vi "Demo Main_before_improvements.vi"() -> ()   [LabVIEW 2022 SP3]
uses:
  C:/Users/Public/OneDrive/Desktop/PMT program/SampleCodeLabView/Kinesis_with_LabVIEW_Examples_LV12 - v3/Thorlabs.MotionControl.Controls.dll
  Kinesis_with_LabVIEW_Examples_LV12 - v3/Thorlabs.MotionControl.Controls.dll
  C:/Users/Public/OneDrive/Desktop/PMT program/SampleCodeLabView/Kinesis_with_LabVIEW_Examples_LV12 - v3/ThorLabs.MotionControl.KCube.DCServoCLI.dll
  Kinesis_with_LabVIEW_Examples_LV12 - v3/ThorLabs.MotionControl.KCube.DCServoCLI.dll
  <vilib>/Utility/file.llb/Write Delimited Spreadsheet (I64).vi
  <vilib>/Utility/file.llb/Write Delimited Spreadsheet (string).vi
  <vilib>/Analysis/NI_AALBase.lvlib
  <vilib>/Utility/file.llb/Write Delimited Spreadsheet (DBL).vi
  Logo.ctl
panel:
  out "ESD":i32=10000 caption="Steps\nAdded/Removed"
  in  "ES":i32 caption="Add /Remove \nSteps"
  out "Sweep Graph":u32[](graph)
  out "SM":i32 caption="Sweep\nMean"
  out "SN":i32 caption="Current Sweep Iteration"
  out "SND":i32 caption="Total No. of Sweeps"
  in  "Auto-Sweep":bool
  in  "P8":bool
  out "PC":i32 caption="Current \nPosition"
  out "WTD":i32=10000 caption="Wait Time (ms)\nRead Data"
  out "EPD":i32 caption="End Position\nRead Data"
  out "SPD":i32 caption="Start Position\nRead Data"
  out "SSD":i32 caption="Step Size\nRead Data"
  in  "SP":i32 caption="Start Position (degrees)\n Set Data"
  in  "WT":i32=10000 caption="Wait Time (ms)\n Set Data"
  in  "EP":i32 caption="End Position (degrees)\n Set Data"
  in  "P7":bool
  in  "SS":i32 caption="Step Size (degrees)\nSet Data"
  in  "Motor Controller\nSerialNumber":string="27261255"
  in  "KCubeDCServoControl":refnum<k24>(container)
  in  "Export":bool
  out "DB":u32[](array[numeric])
  out "OVL":bool caption="LED ON : Over Rang Data"
  out "OLD":i32
  out "GN":i32 caption="Gate Number"
  in  "Correction":bool
  in  "Logo":T1
  out "Graph":u32[](graph)
  in  "Stop":bool
  in  "Start":bool
  in  "P6":bool
  out "RND":i32 caption="Read Number\nRead Data"
  in  "P5":bool
  in  "RN":i32=100 caption="Read Number\nSet Data"
  out "PowerD":i32 caption="Power\nRead Data"
  out "ITD":i32 caption="Internal Time\nRead Data"
  in  "P4":bool
  in  "P3":bool
  in  "IT":i32=100 caption="Internal Time\nSet Data"
  in  "P2":bool
  out "Handle Number":i32
  in  "P1":bool caption="Switch\nPower OFF/Power ON"
  in  "EXIT":bool
  # "pmt serial: 30430219"
  # "data array isn't being emptied after each sweep...?"
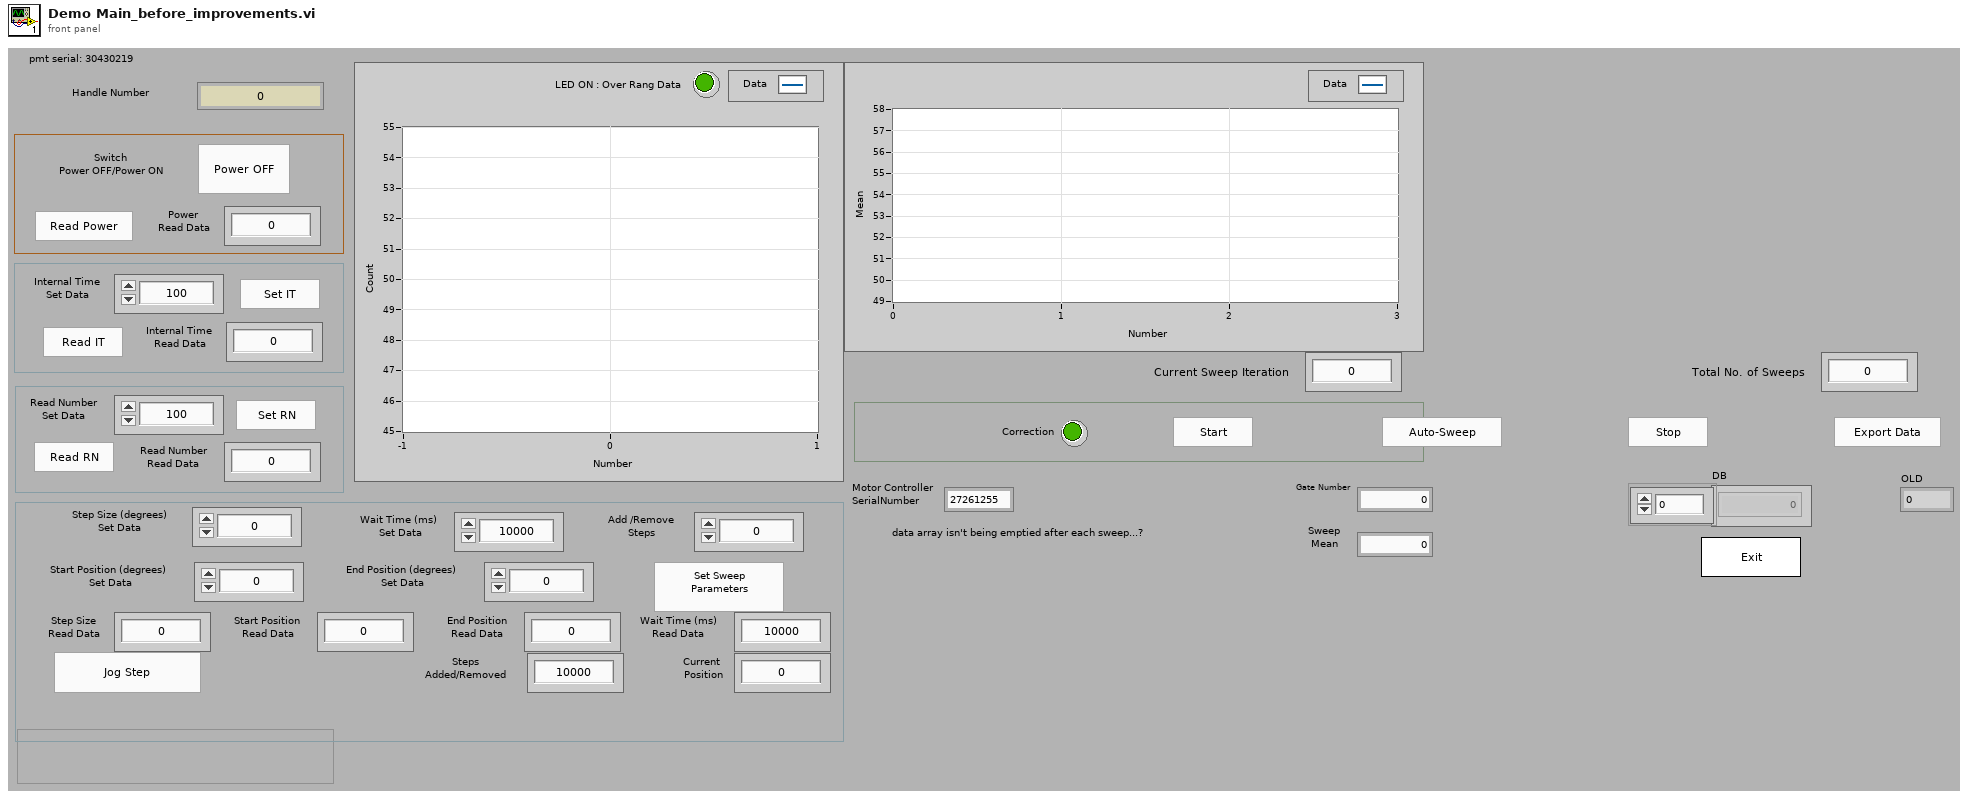
[diagram p1: front panel]
types:
  T1 = typedef "Logo.ctl" = bool
  T2 = enum8{"Enabled", "Disabled", "Disabled and Grayed Out"}
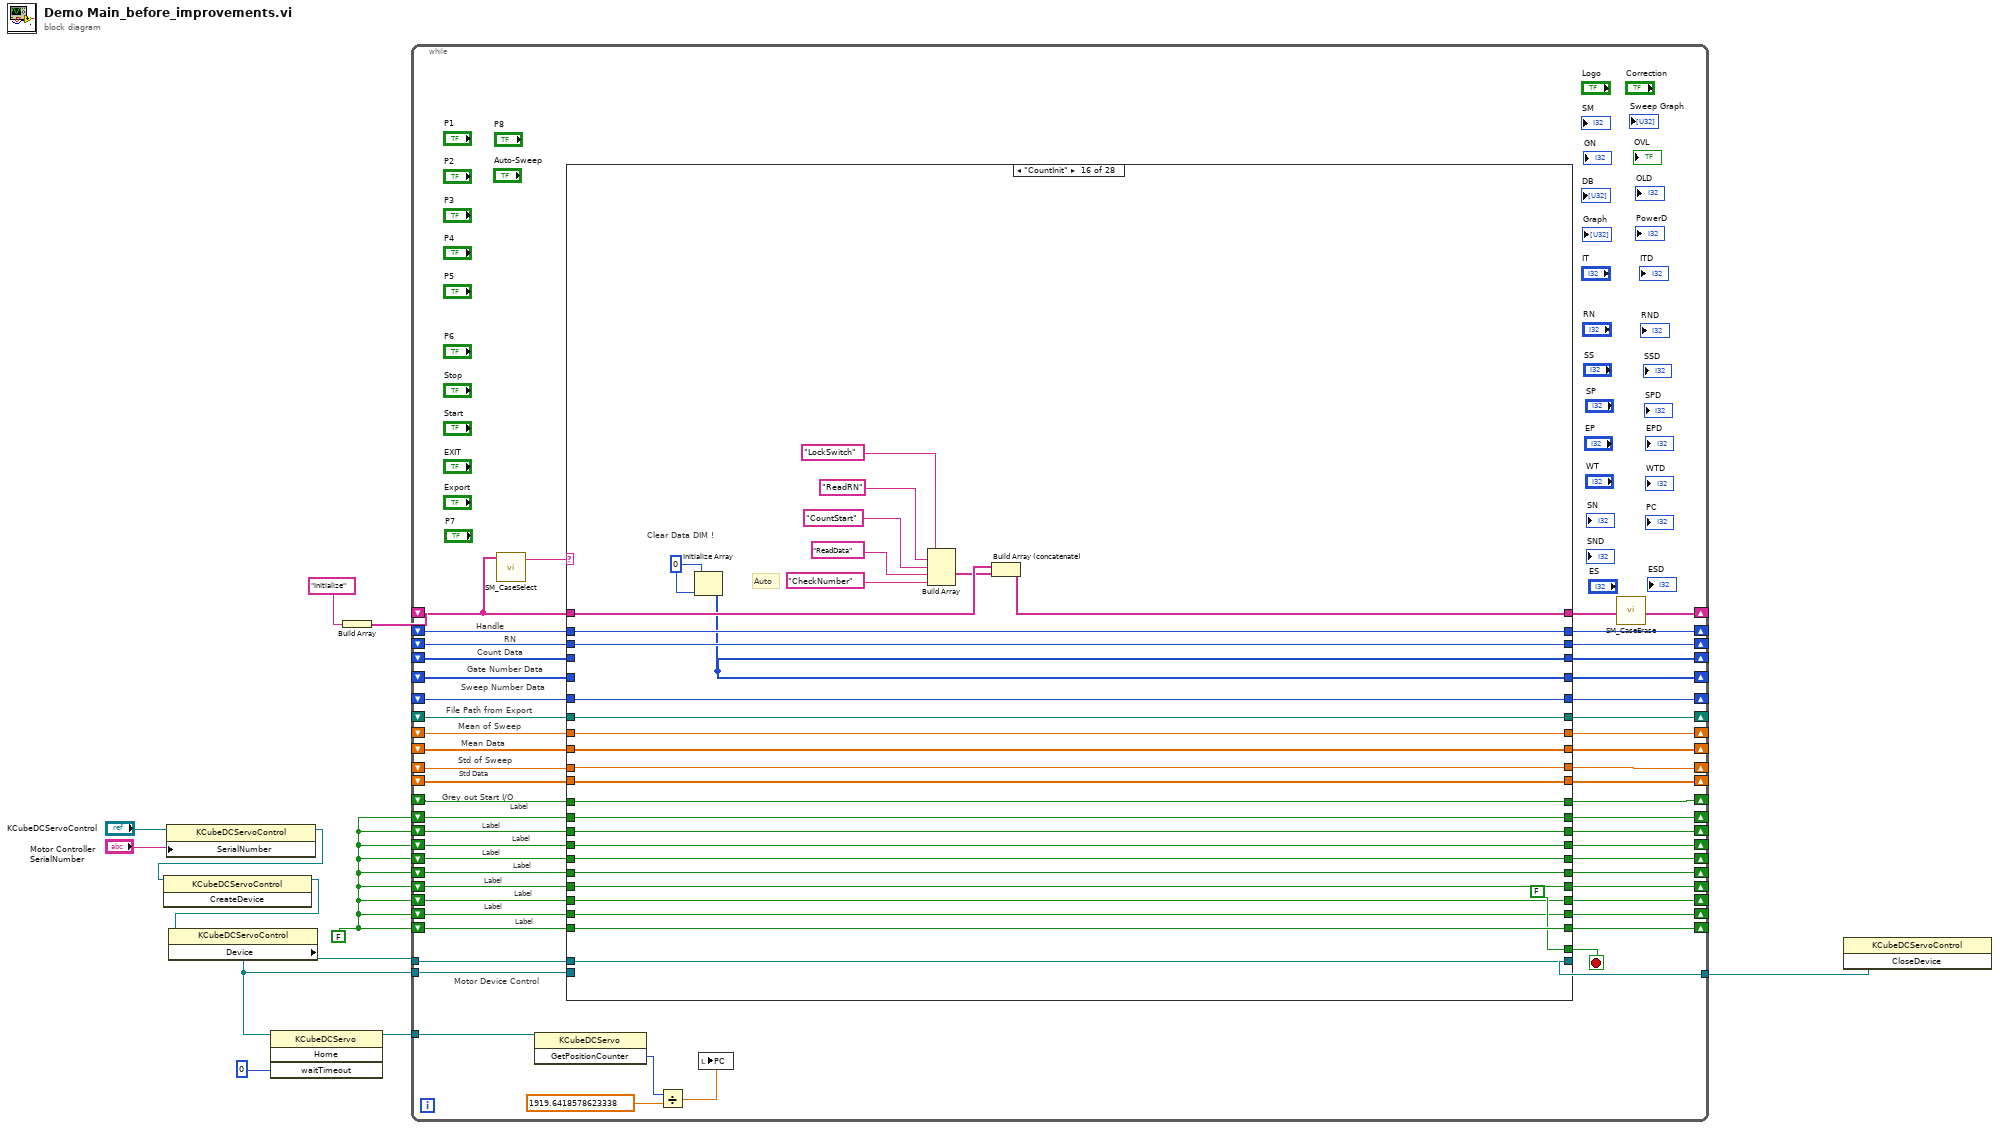
[diagram p0: block diagram]
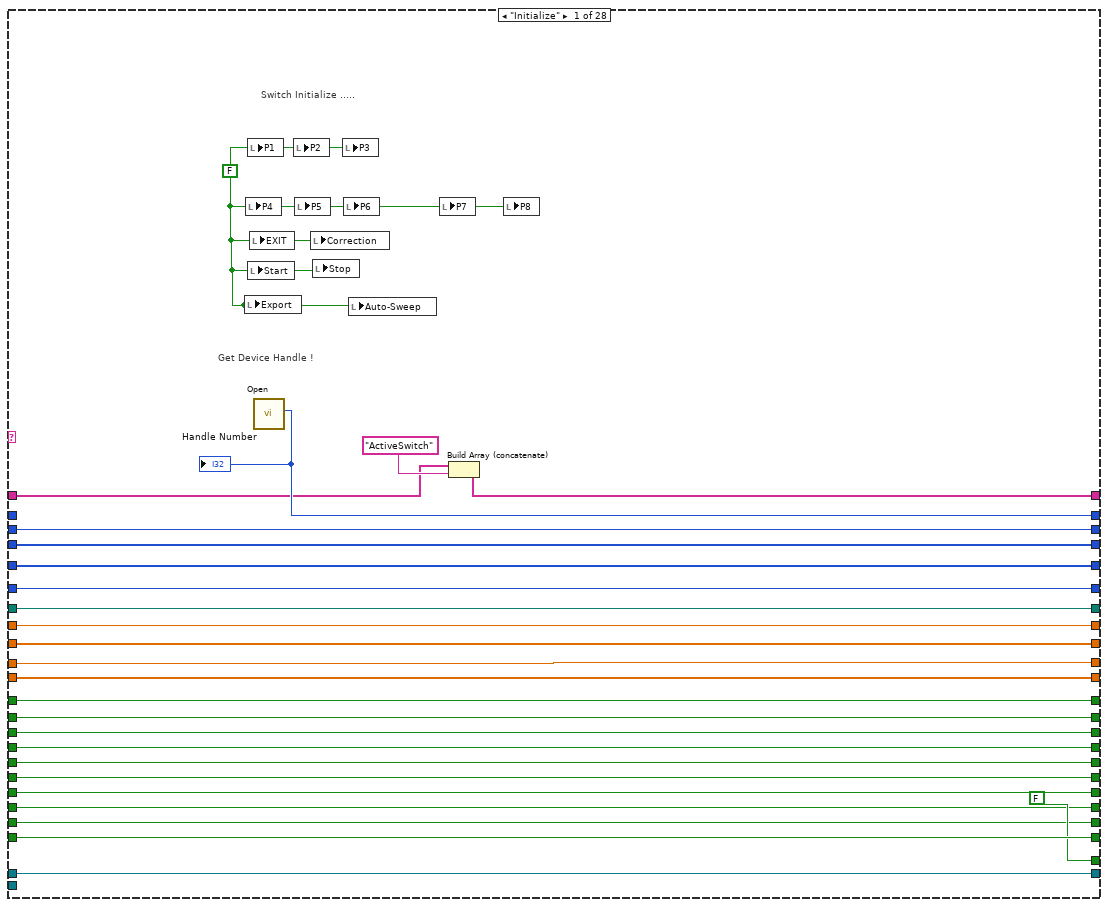
[diagram p2: hidden frame]
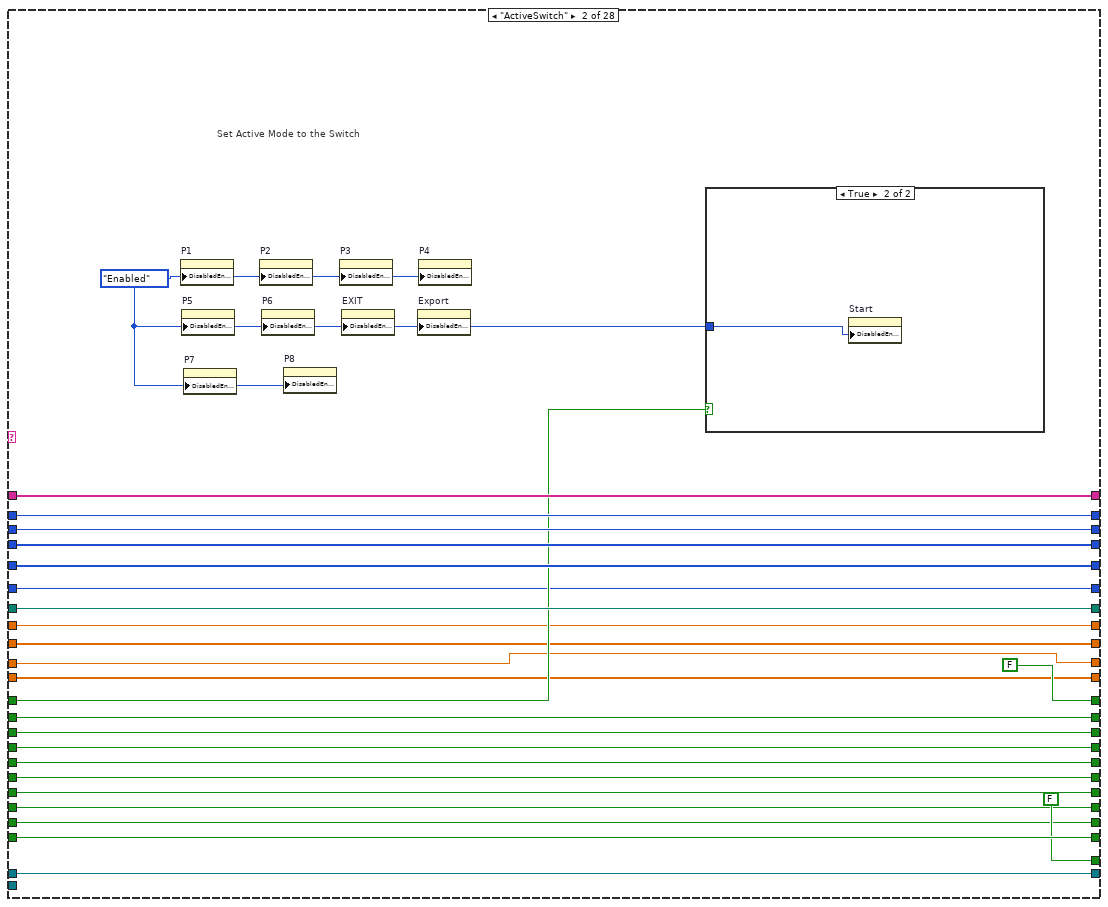
[diagram p3: hidden frame]
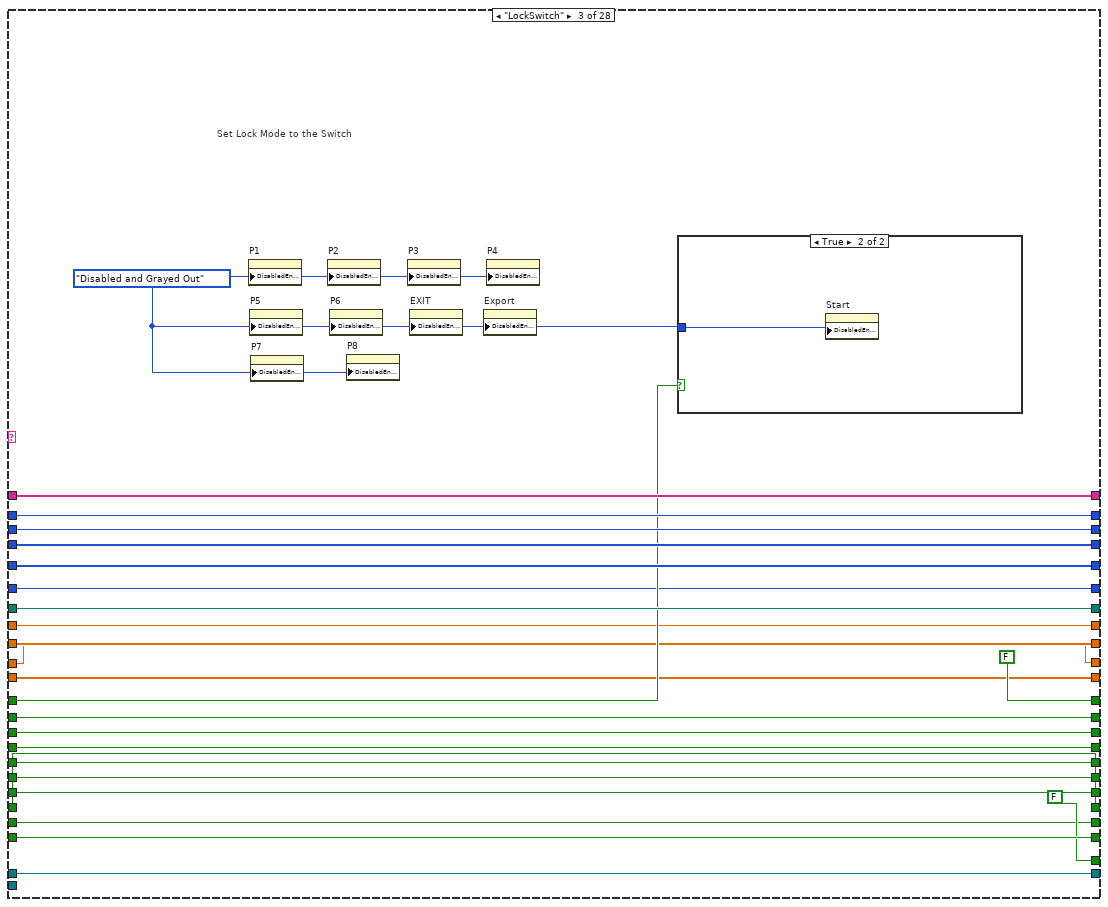
[diagram p5: hidden frame]
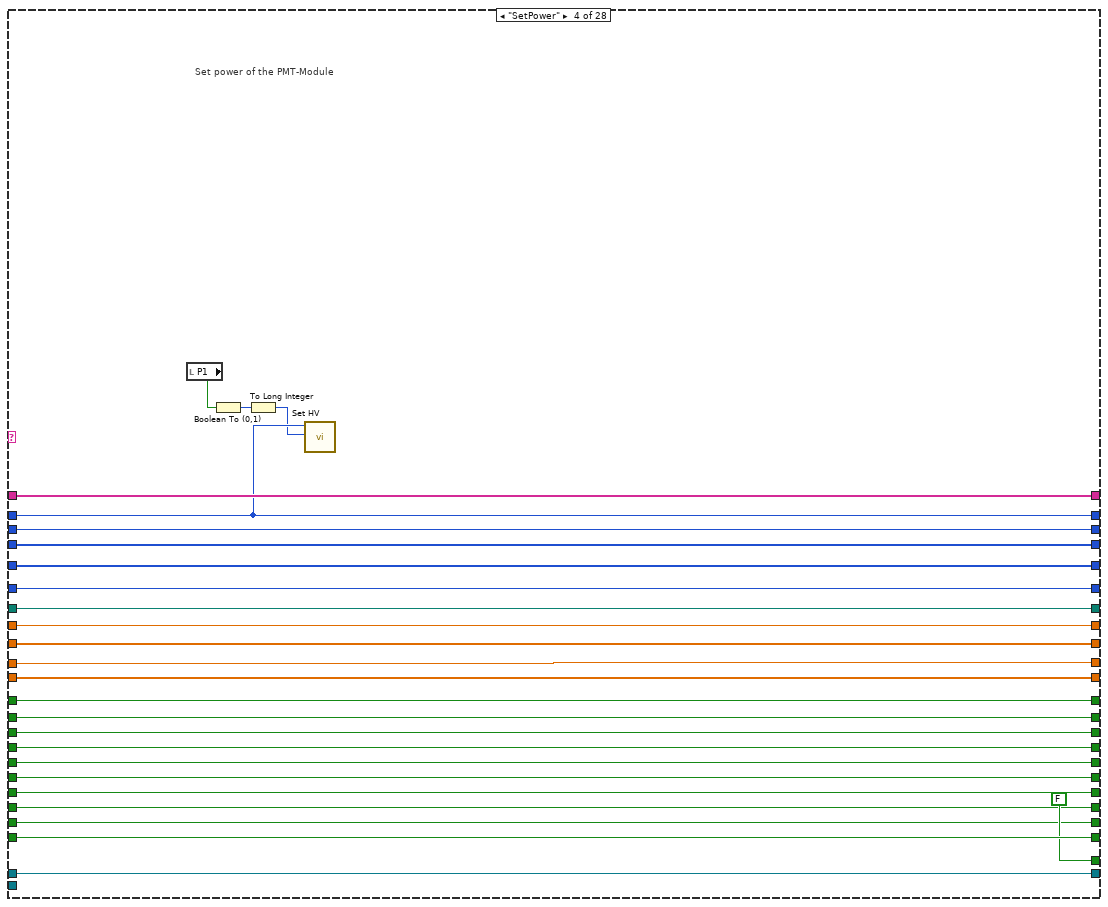
[diagram p7: hidden frame]
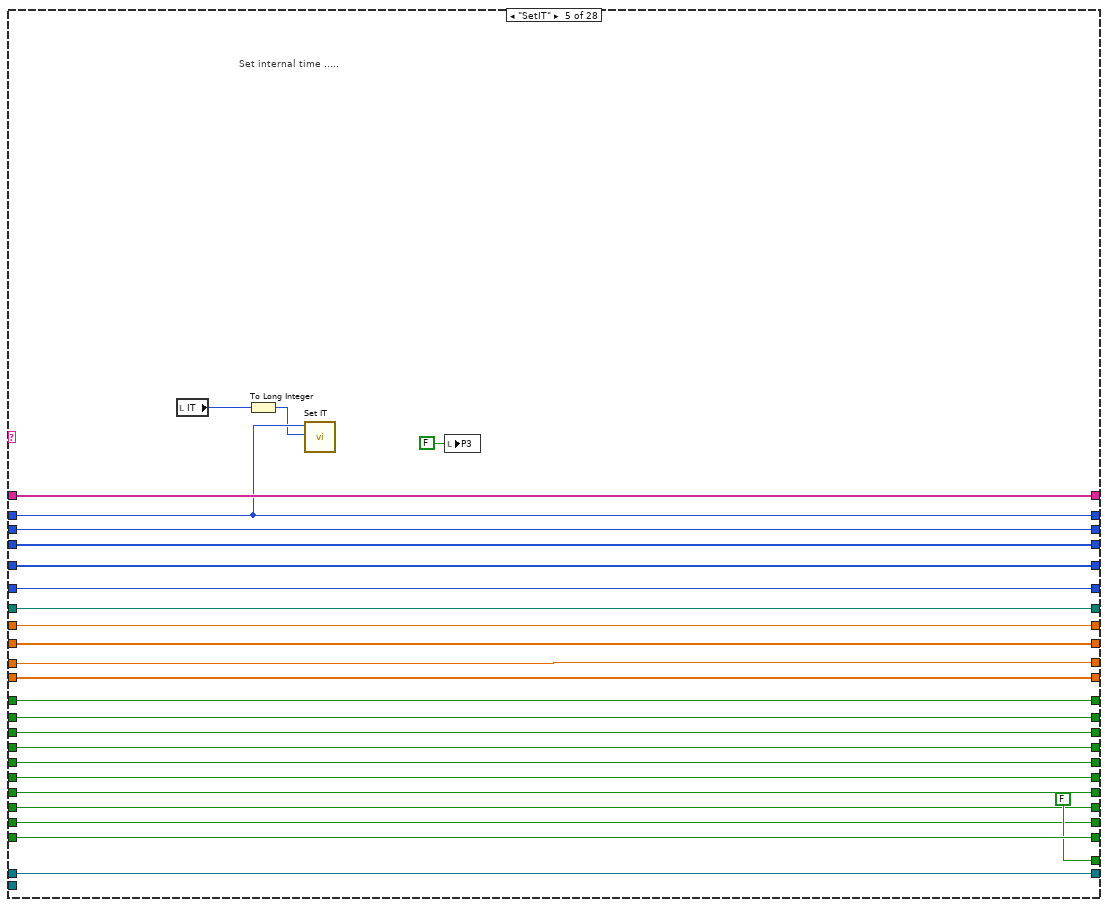
[diagram p8: hidden frame]
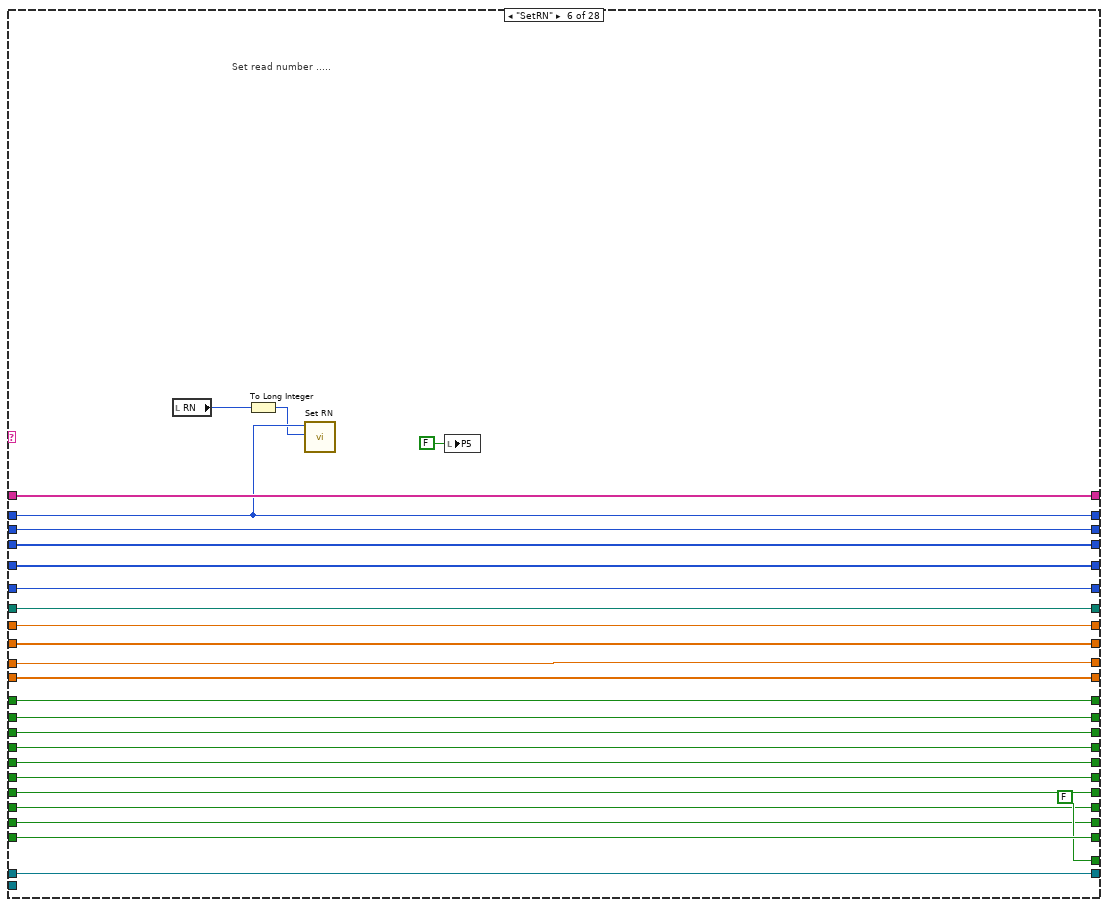
[diagram p9: hidden frame]
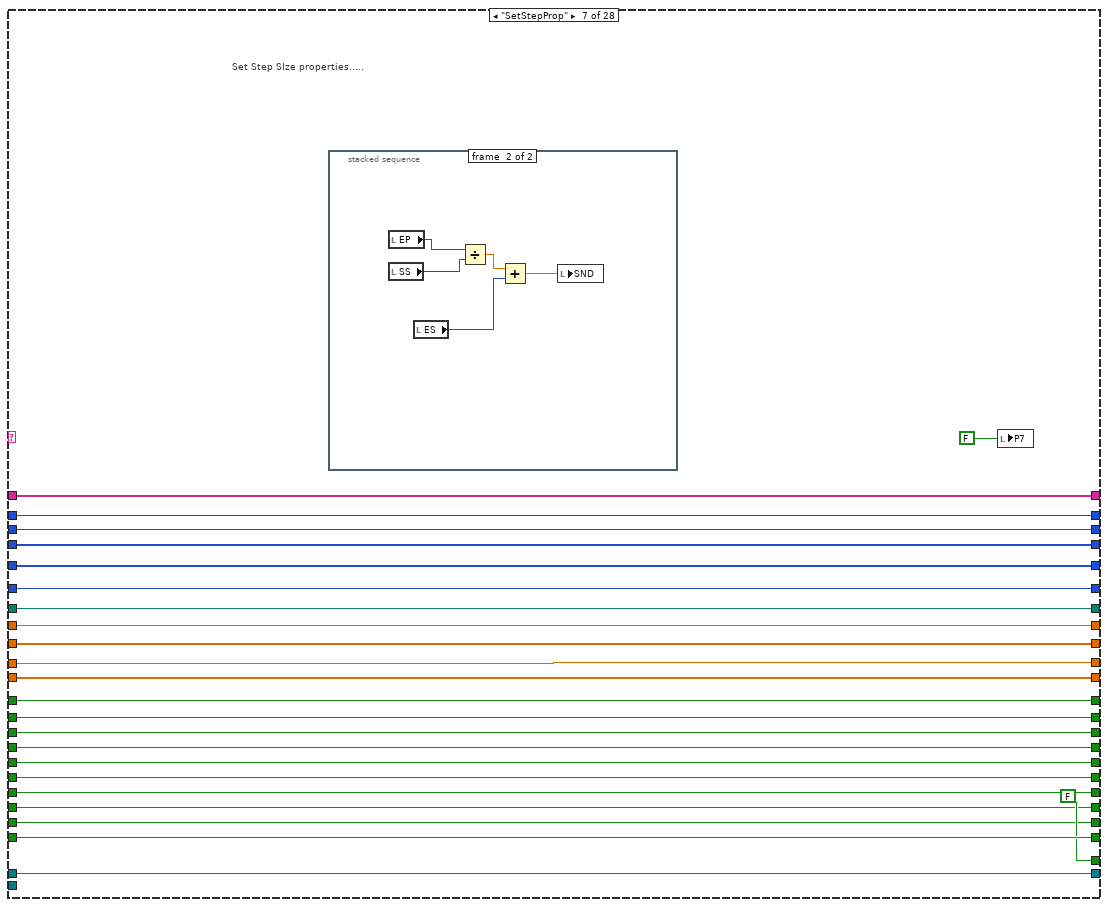
[diagram p10: hidden frame]
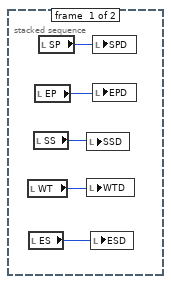
[diagram p11: hidden frame]
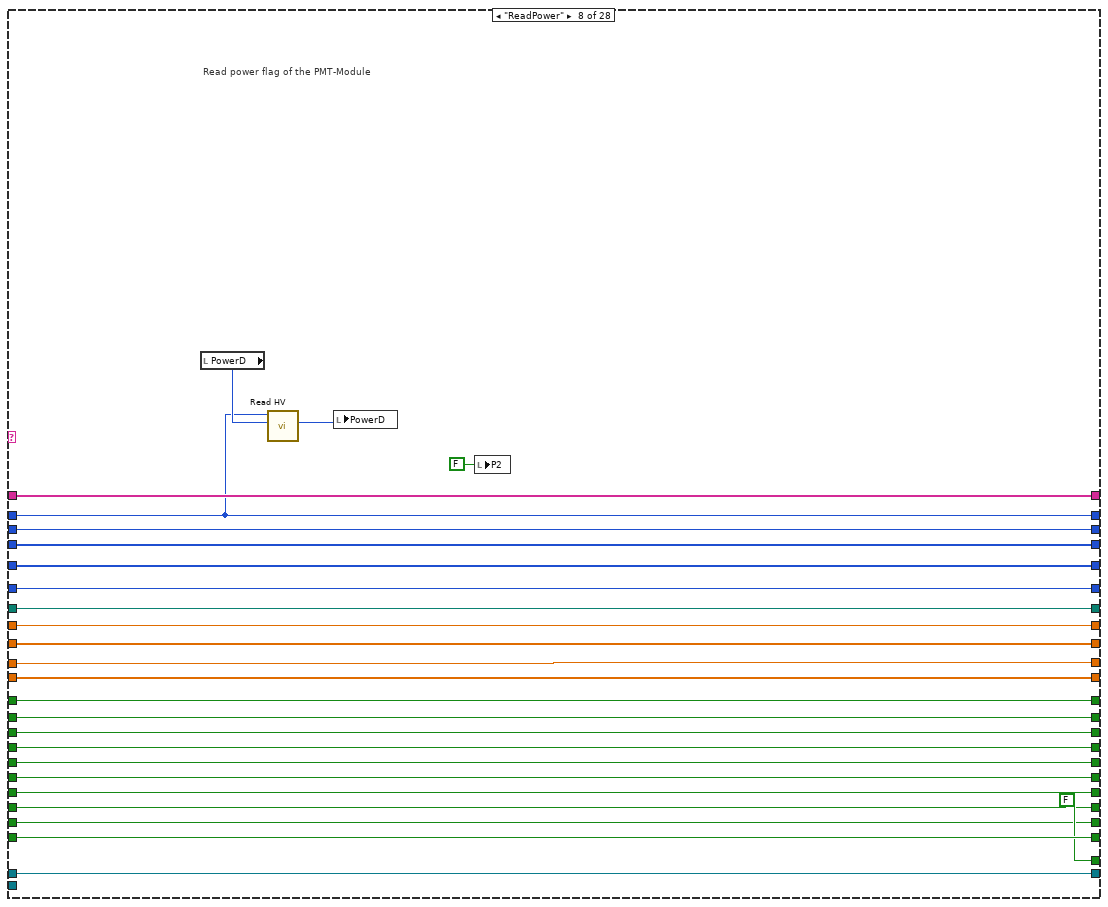
[diagram p12: hidden frame]
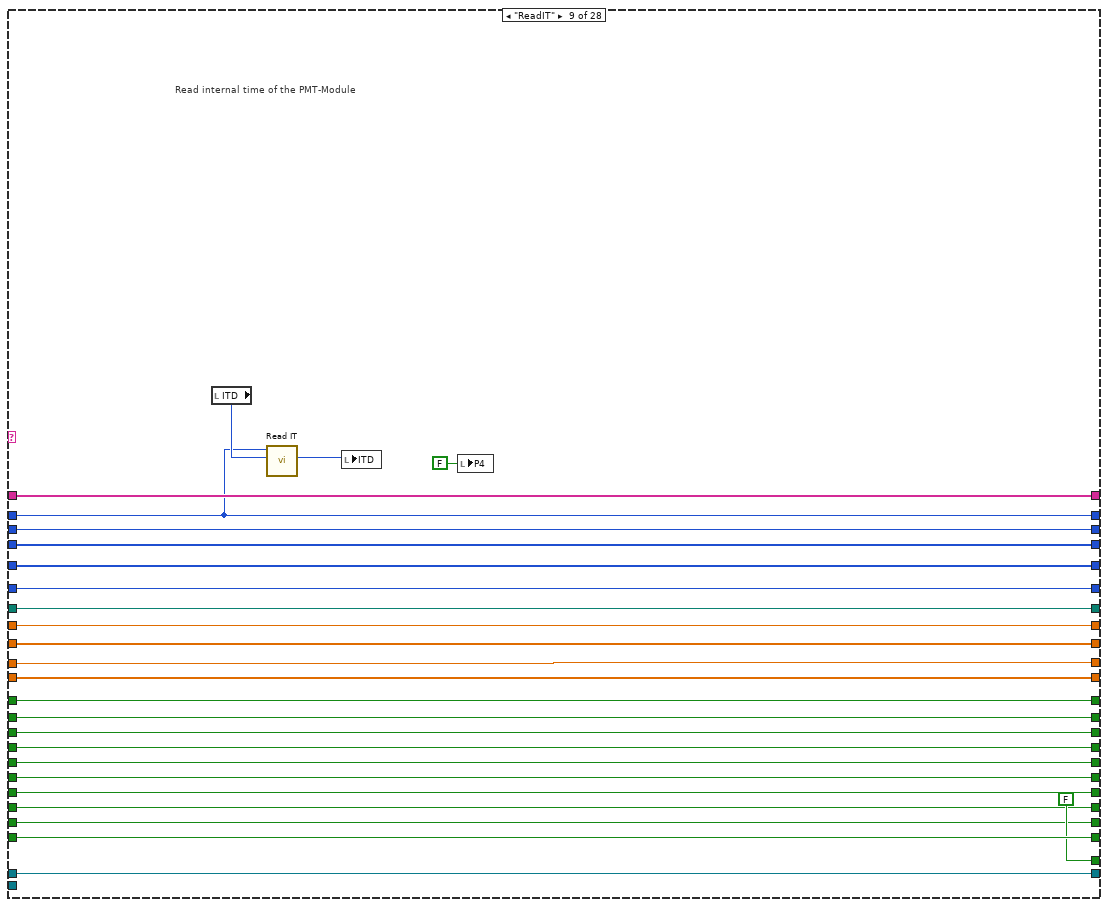
[diagram p13: hidden frame]
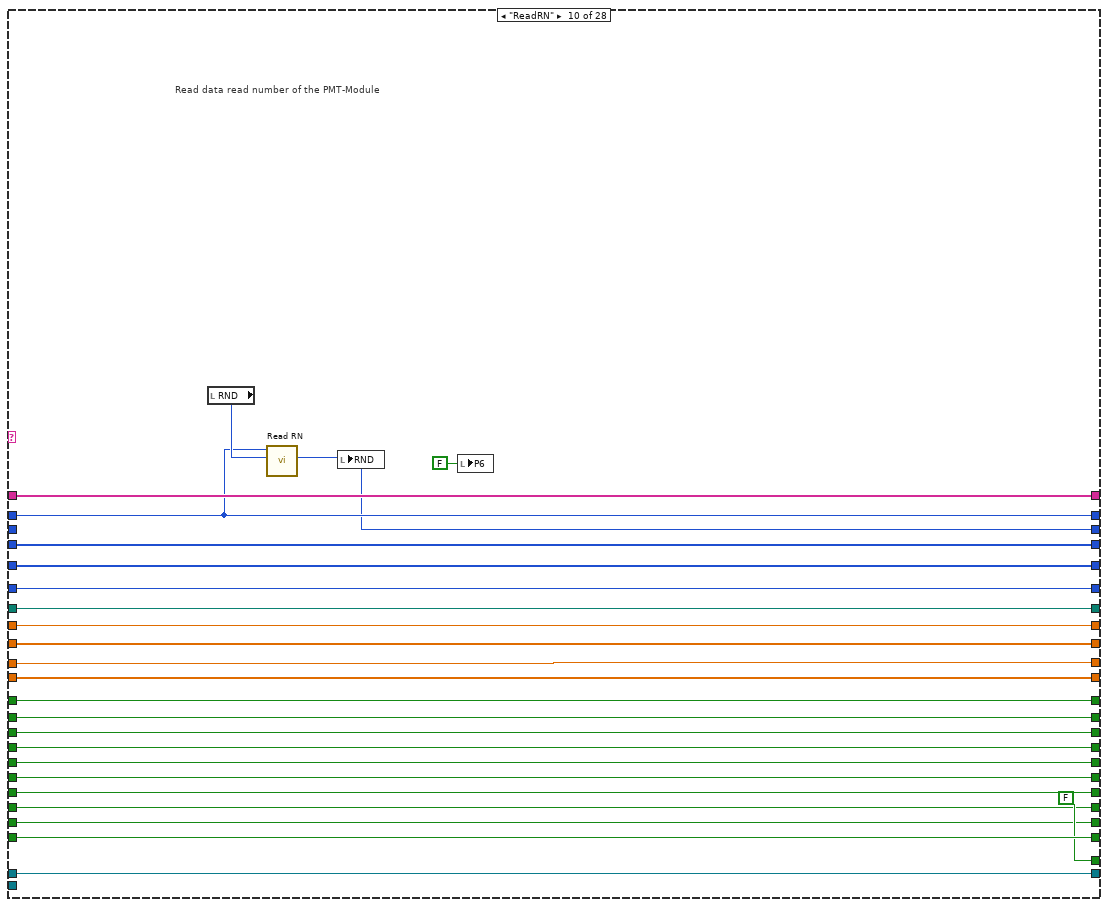
[diagram p14: hidden frame]
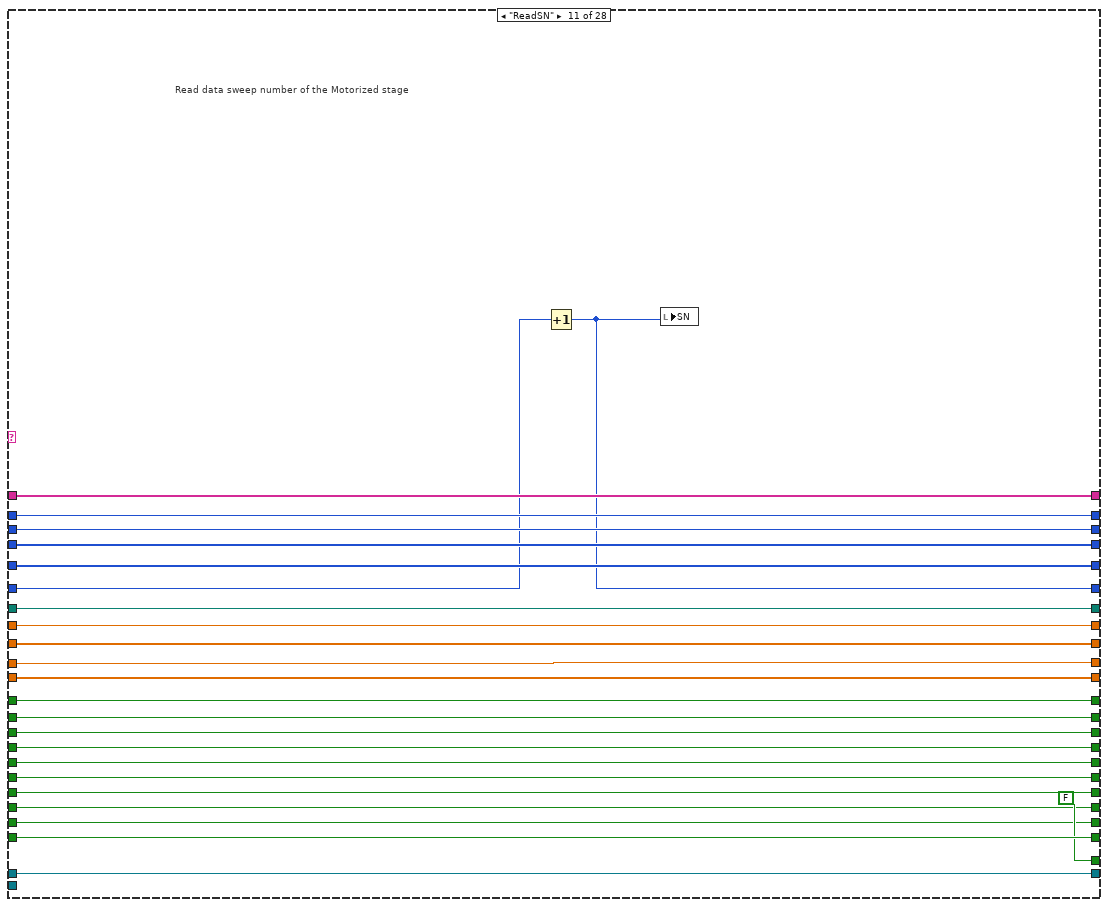
[diagram p15: hidden frame]
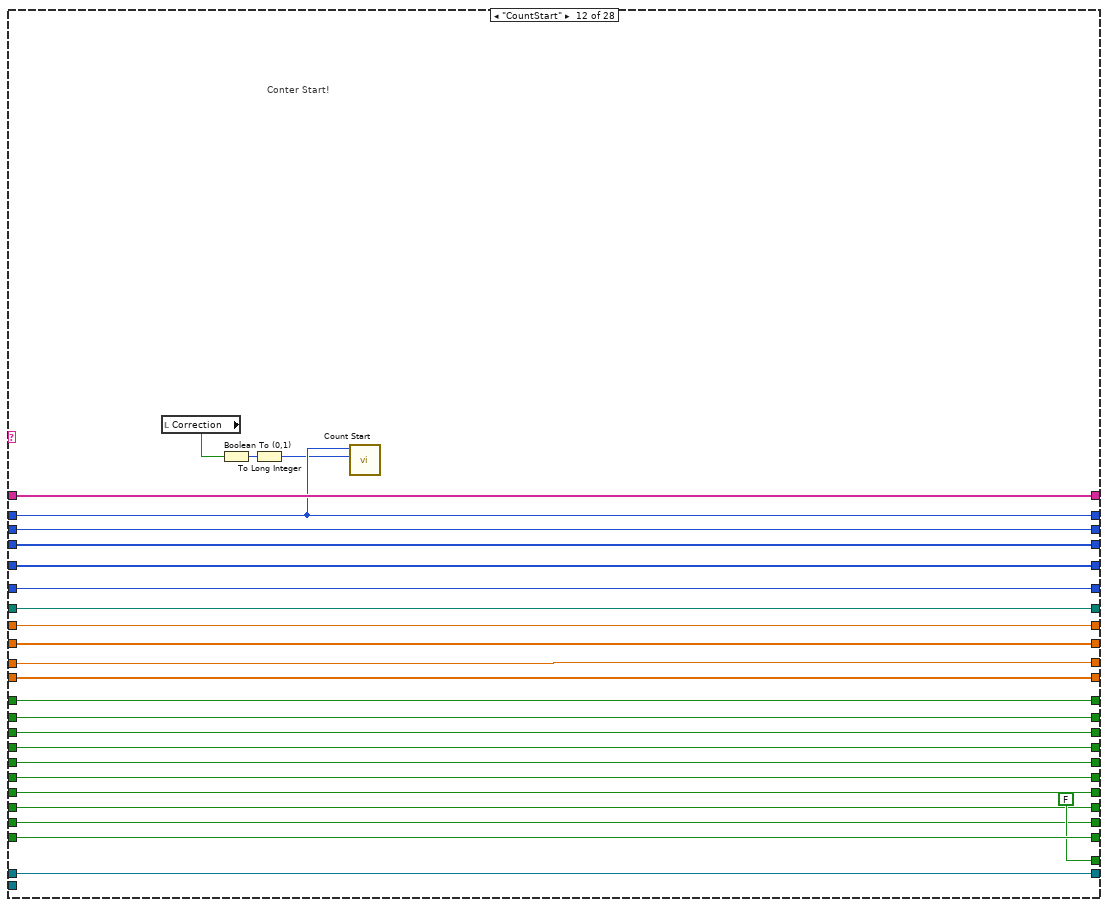
[diagram p16: hidden frame]
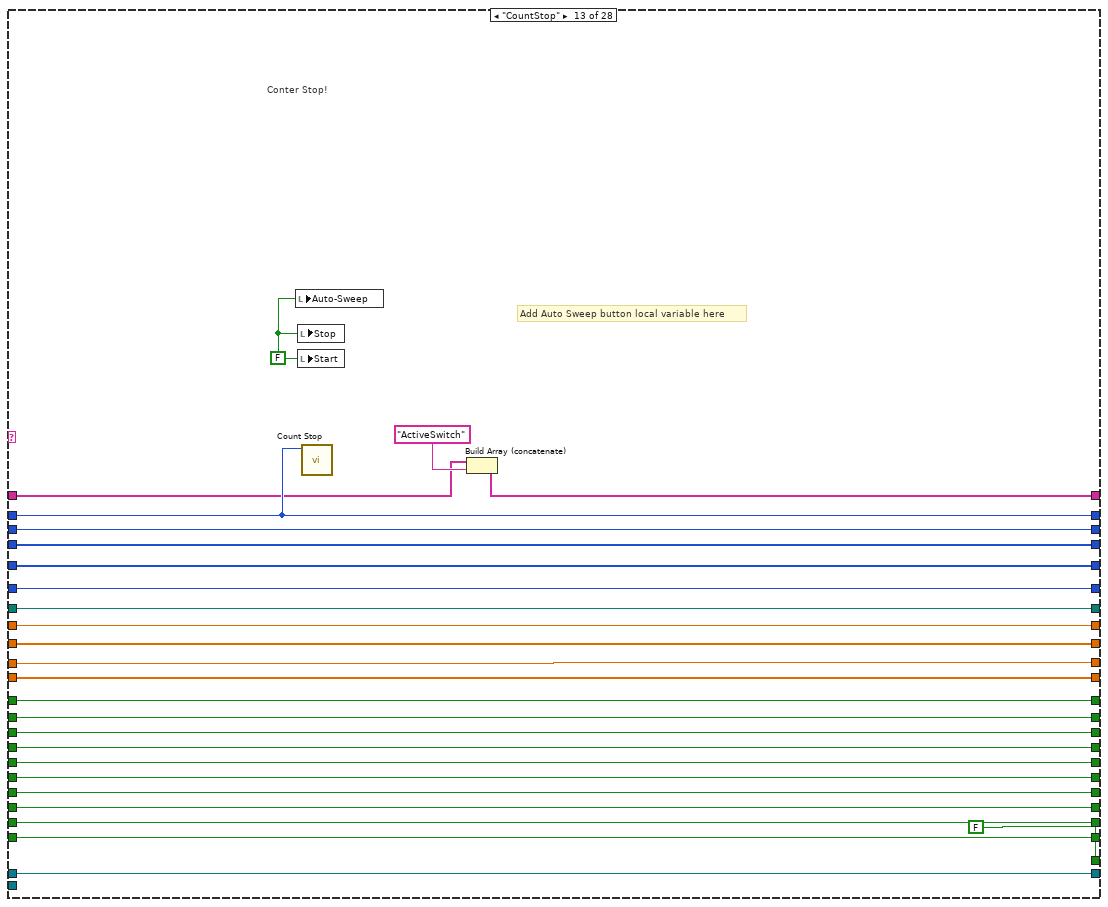
[diagram p17: hidden frame]
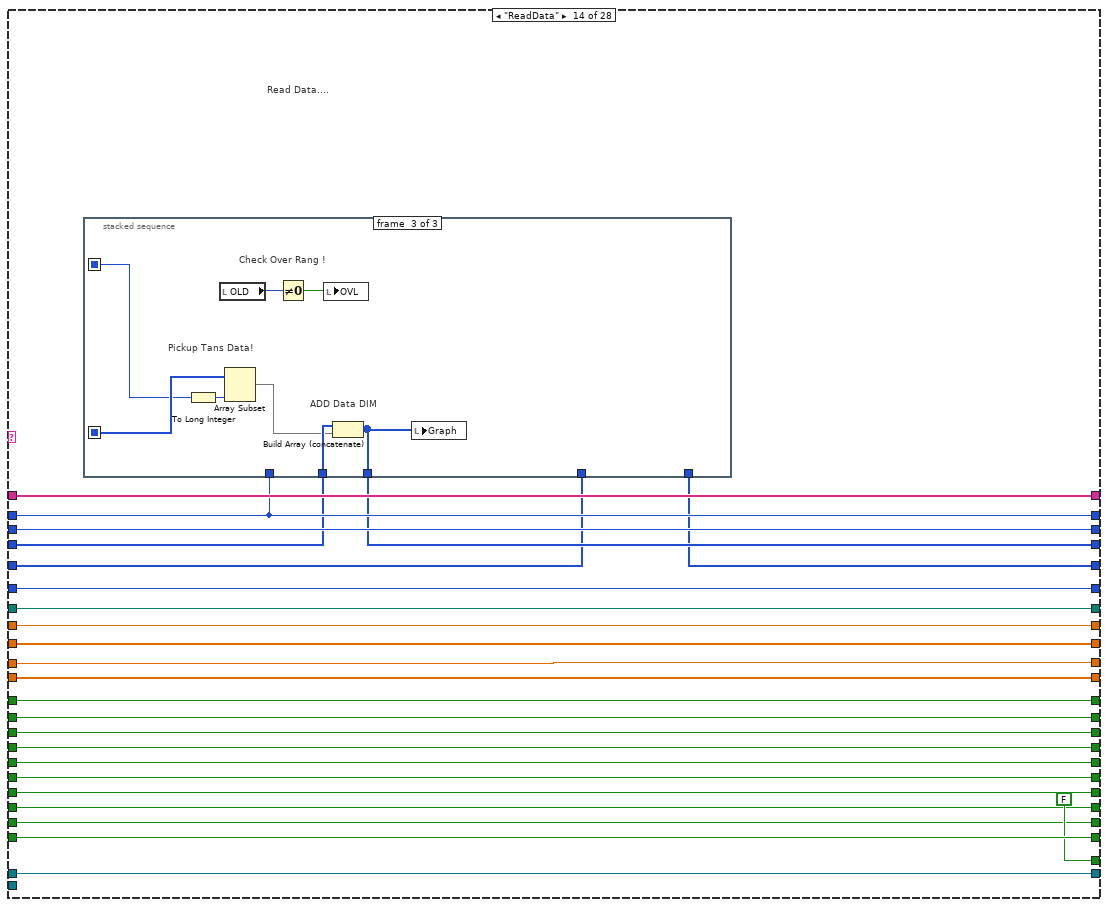
[diagram p18: hidden frame]
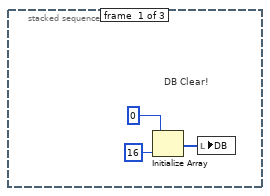
[diagram p19: hidden frame]
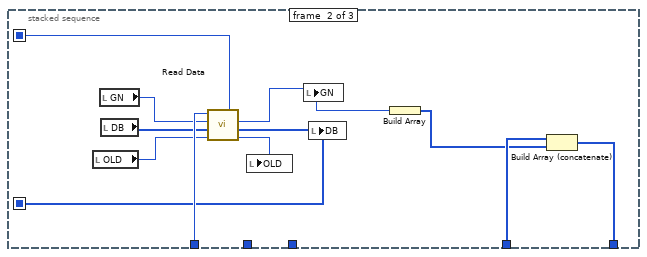
[diagram p20: hidden frame]
diagram:
  w10 = FALSE
  n1 = property class="KCubeDCServoControl"(reference="KCubeDCServoControl", "SerialNumber"="Motor Controller\nSerialNumber") -> (reference out=w8:refnum<k24>)  [unwired: 1 in, 1 out]
  n2 = invoke class="KCubeDCServoControl" method="CreateDevice"(reference=w8) -> (reference out=w1:refnum<k24>)  [unwired: 2 in, 2 out]
  n3 = property class="KCubeDCServoControl"(reference=w1) -> (reference out=w5:refnum<k24>, "Device"=w3:refnum<k24>)  [unwired: 1 in, 1 out]
  n4 = invoke class="KCubeDCServo" method="Home"(reference=w3, "waitTimeout"=0) -> (reference out=w2:refnum<k24>)  [unwired: 2 in, 3 out]
  n5 = Build Array("Initialize") -> (w11:string[])
  n6 = while {
    shift-right: [w47] -> _
    shift-left: w10 -> [w48]
    shift-right: [w49] -> _
    shift-left: w10 -> [w50]
    shift-right: [w51] -> _
    shift-left: w10 -> [w52]
    shift-right: [w53] -> _
    shift-left: w10 -> [w54]
    shift-right: [w55] -> _
    shift-left: _ -> [w56]
    shift-right: [w57] -> _
    shift-left: _ -> [w58]
    shift-right: [w59] -> _
    shift-left: _ -> [w60]
    shift-right: [w45] -> _
    shift-left: w10 -> [w46]
    shift-right: [w63] -> _
    shift-left: w10 -> [w64]
    shift-right: [w42] -> _
    shift-left: w11 -> [w61]
    shift-right: [w40] -> _
    shift-left: w10 -> [w41]
    shift-right: [w38] -> _
    shift-left: w10 -> [w39]
    shift-right: [w37] -> _
    shift-left: w10 -> [w36]
    tunnel: w5 -> [w33]
    tunnel: [w32] -> w6
    shift-right: [w35] -> _
    shift-left: _ -> [w34]
    tunnel: w3 -> [w31]
    shift-right: [w30] -> _
    shift-left: _ -> [w29]
    shift-right: [w28] -> _
    shift-left: _ -> [w27]
    tunnel: w2 -> [w26]
    shift-right: [w24] -> _
    shift-left: _ -> [w25]
    shift-right: [w23] -> _
    shift-left: _ -> [w22]
    shift-right: [w21] -> _
    shift-left: _ -> [w20]
    shift-right: [w13] -> _
    shift-left: _ -> [w16]
    shift-right: [w14] -> _
    shift-left: _ -> [w15]
    stop <- w44 stop-if-true
    # "Std Data"
    # "Std of Sweep"
    # "Mean Data"
    # "Mean of Sweep"
    # "Sweep Number Data"
    # "Grey out Start I/O"
    # "Motor Device Control"
    # "File Path from Export"
    # "Gate Number Data"
    # "Label"
    # "Label"
    # "Label"
    # "Label"
    # "Label"
    # "Label"
    # "Label"
    # "Label"
    # "Label"
    # "Count Data"
    # "RN"
    # "Handle"
    n7 = call "SM_CaseSelect.vi"("Input"=w61) -> ("Case"=w62:string)  [unwired: 10 out]
    n8 = invoke class="KCubeDCServo" method="GetPositionCounter"(reference=w26) -> ("GetPositionCounter"=w18:i32)  [unwired: 2 in, 2 out]
    n9 = case shown="\"CountInit\"" w62 {
      selector: w62 -> [_ _ _ _ _ _ _ _ _ _ _ _ _ _ _ _ _ _ _ _ _ _ _ _ _ _ w996 _]
      tunnel: w64 -> [w90 w115 w141 w168 w194 w220 w244 w280 w306 w331 w355 w381 w407 w432 w478 w511 w539 w581 w621 w692 w746 w802 w834 w858 w892 w941 w1014 w1037]
      tunnel: [w90 w115 w141 w168 w194 w220 w244 w280 w306 w331 w355 w381 w407 w432 w478 w511 w539 w581 w621 w692 w746 w802 w834 w858 w892 w941 w1014 w1037] -> w63
      tunnel: w61 -> [w76 w114 w140 w167 w193 w219 w243 w279 w305 w330 w354 w380 w393 w431 w477 w499 w517 w568 w609 w703 w757 w813 w826 w871 w905 w929 w1013 w1036]
      tunnel: [w75 w114 w140 w167 w193 w219 w243 w279 w305 w330 w354 w380 w392 w431 w477 w498 w516 w569 w610 w703 w757 w813 w825 w871 w905 w926 w1013 w1036] -> w43
      tunnel: w60 -> [_ w102 w128 w155 w181 w207 w231 w266 w292 w318 w343 w368 w395 w420 w466 w500 w528 w571 w611 w702 w756 w812 w846 w870 w904 w940 w1012 w1024]
      tunnel: [w78 w102 w128 w155 w181 w207 w231 w266 w292 w318 w343 w368 w395 w420 w466 w500 w528 w571 w611 w702 w756 w812 w846 w870 w904 w940 w1012 w1024] -> w59
      tunnel: w58 -> [w89 w113 w139 w166 w192 w218 w242 w278 w304 _ w336 w379 w406 w430 w476 w510 w538 w566 w607 w701 w755 w811 w845 w869 w903 w939 w1011 w1035]
      tunnel: [w89 w113 w139 w166 w192 w218 w242 w278 w304 w316 w336 w379 w406 w430 w476 w510 w538 w566 w607 w701 w755 w811 w845 w869 w903 w939 w1011 w1035] -> w57
      tunnel: w56 -> [w88 w112 w138 w165 w191 w217 w241 w277 w303 w329 w353 w378 w405 w419 w461 _ _ w562 w605 w677 w731 w787 w844 w868 w902 w925 w1010 w1034]
      tunnel: [w88 w112 w138 w165 w191 w217 w241 w277 w303 w329 w353 w378 w405 w418 w461 w490 w526 w562 w605 w677 w731 w787 w844 w868 w902 w925 w1010 w1034] -> w55
      tunnel: w54 -> [w87 w111 w137 w164 w190 w216 w240 w276 w302 w328 w352 w377 w404 w429 w475 w509 w537 w580 w620 w700 w754 w810 w842 w866 w900 w938 w1009 w1033]
      tunnel: [w87 w111 w137 w164 w190 w216 w240 w276 w302 w328 w352 w377 w404 w429 w475 w509 w537 w580 w620 w700 w754 w810 w842 w866 w900 w938 w1009 w1033] -> w53
      tunnel: w52 -> [w86 w110 w136 w163 w189 w215 w239 w275 w301 w327 w351 w376 w403 w428 w474 w508 w536 w579 w619 w699 w753 w809 w841 w865 w899 w937 w1008 w1032]
      tunnel: [w86 w110 w136 w163 w189 w215 w239 w275 w301 w327 w351 w376 w403 w428 w474 w508 w536 w579 w619 w699 w753 w809 w841 w865 w899 w937 w1008 w1032] -> w51
      tunnel: w50 -> [w85 w109 w135 w162 w188 w214 w238 w274 w300 w326 w350 w375 w402 w427 w473 w507 w535 w578 w618 w698 w752 w808 w840 w864 w898 w936 w1007 w1031]
      tunnel: [w85 w109 w135 w162 w188 w214 w238 w274 w300 w326 w350 w375 w402 w427 w473 w507 w535 w578 w618 w698 w752 w808 w840 w864 w898 w936 w1007 w1031] -> w49
      tunnel: w48 -> [w84 w108 w134 w161 w187 w213 w237 w273 w299 w325 w349 w374 w401 w426 w472 w506 w534 w577 w617 w697 w751 w807 w839 w863 w897 w935 w1006 w1030]
      tunnel: [w84 w108 w134 w161 w187 w213 w237 w273 w299 w325 w349 w374 w401 w426 w472 w506 w534 w577 w617 w697 w751 w807 w839 w863 w897 w935 w1006 w1030] -> w47
      tunnel: w46 -> [w83 w107 w133 w160 w186 w212 w236 w272 w298 w324 w348 w373 w400 w425 w471 w505 w533 w576 w616 w696 w750 w806 w838 w862 w896 w934 w1005 w1029]
      tunnel: [w83 w107 w133 w160 w186 w212 w236 w272 w298 w324 w348 w373 w400 w425 w471 w505 w533 w576 w616 w696 w750 w806 w838 w862 w896 w934 w1005 w1029] -> w45
      tunnel: [FALSE FALSE FALSE FALSE FALSE FALSE FALSE FALSE FALSE FALSE FALSE FALSE FALSE FALSE FALSE FALSE FALSE FALSE FALSE FALSE FALSE FALSE FALSE FALSE FALSE FALSE FALSE TRUE] -> w44
      tunnel: w41 -> [w79 w103 w129 w156 w182 w208 w232 w268 w294 w320 w344 w369 w396 w421 w467 w501 w529 w572 w612 w695 w749 w805 w837 w861 w895 w930 w1001 w1025]
      tunnel: [w79 w103 w129 w156 w182 w208 w232 w268 w294 w320 w344 w369 w396 w421 w467 w501 w529 w572 w612 w695 w749 w805 w837 w861 w895 w930 w1001 w1025] -> w40
      tunnel: w39 -> [w81 w105 w131 w158 w184 w210 w234 w270 w296 w322 w346 w371 w398 w423 w469 w503 w531 w574 w614 w694 w748 w804 w836 w860 w894 w932 w1003 w1027]
      tunnel: [w81 w105 w131 w158 w184 w210 w234 w270 w296 w322 w346 w371 w398 w423 w469 w503 w531 w574 w614 w694 w748 w804 w836 w860 w894 w932 w1003 w1027] -> w38
      tunnel: [w80 w104 w130 w157 w183 w209 w233 w269 w295 w321 w345 w370 w397 w422 w468 w502 w530 w573 w613 w693 w747 w803 w835 w859 w893 w931 w1002 w1026] -> w37
      tunnel: w36 -> [w80 w104 w130 w157 w183 w209 w233 w269 w295 w321 w345 w370 w397 w422 w468 w502 w530 w573 w613 w693 w747 w803 w835 w859 w893 w931 w1002 w1026]
      tunnel: [w74 w101 w127 w151 w177 w203 w230 w263 w289 w315 w342 w364 w391 w417 w460 w490 w526 w561 w604 w672 w726 w782 w843 w867 w901 w924 w995 w1023] -> w35
      tunnel: w34 -> [w74 w101 w127 w151 w177 w203 w230 w263 w289 w315 w342 w364 w391 w416 w460 _ _ w561 w604 w672 w726 w782 w843 w867 w901 w924 w995 w1023]
      tunnel: w33 -> [w73 w100 w126 w150 w176 w202 w229 w262 w288 w314 w341 w363 w390 w415 w465 w489 w525 w560 w603 w674 w728 w784 w833 w857 w891 w923 w994 w1022]
      tunnel: [w73 w100 w126 w150 w176 w202 w229 w262 w288 w314 w341 w363 w390 w415 w465 w489 w525 w560 w603 w674 w728 w784 w833 w857 w891 w923 w994 w1022] -> w32
      tunnel: w31 -> [_ _ _ _ _ _ _ _ _ _ _ _ _ _ _ _ _ _ _ _ _ _ _ w854 w888 _ _ _]
      tunnel: [w72 w99 w125 w149 w175 w201 w227 w261 w287 w313 w340 w362 w389 w414 w464 w488 w524 w559 w602 w665 w723 w778 w822 w855 w889 w922 w993 w1021] -> w30
      tunnel: w29 -> [w72 w99 w125 w149 w175 w201 w227 w261 w287 w313 w340 w362 w389 w414 w464 w488 w524 w559 w602 w665 w719 w776 _ w855 w889 w922 w993 w1021]
      tunnel: [w71 FALSE FALSE w148 w174 w200 w226 w260 w286 w312 w339 w361 w388 w413 w463 w487 TRUE w558 w601 w667 w722 w777 w831 w853 w887 w921 w992 w1020] -> w28
      tunnel: w27 -> [w71 w98 w124 w148 w174 w200 w226 w260 w286 w312 w339 w361 w388 w413 w463 w487 _ w558 _ w667 w722 w777 w831 w853 w887 w921 w992 w1020]
      tunnel: w25 -> [w69 w95 w121 w147 w173 w199 w225 w259 w285 w311 w334 w360 w387 w412 w462 w486 w522 w557 w600 w666 w715 w773 _ w849 w886 w920 w991 w1019]
      tunnel: [w69 w95 w121 w147 w173 w199 w225 w259 w285 w311 w335 w360 w387 w412 w462 w486 w522 w557 w600 w666 w715 w773 w823 w849 w886 w920 w991 w1019] -> w24
      tunnel: [w68 w94 w120 w146 w172 w198 w224 w258 w284 w310 w338 w359 w386 w411 w459 w485 w521 w556 w597 w664 w721 w775 w830 w851 w885 w919 w990 w1018] -> w23
      tunnel: w22 -> [w68 w94 w120 w146 w172 w198 w224 w258 w284 w310 w338 w359 w386 w411 w459 w485 w521 w556 w597 w664 _ _ w830 w851 w885 w919 w990 w1018]
      tunnel: [w67 w93 w119 w145 w171 w197 w223 w257 w283 w309 w337 w358 w385 w410 w458 w484 w520 w555 w596 w663 w720 w772 w824 w850 w884 w918 w989 w1017] -> w21
      tunnel: w20 -> [w67 w93 w119 w145 w171 w197 w223 w257 w283 w309 w337 w358 w385 w410 w457 w484 w520 w555 w596 w663 w720 w774 w824 w850 w884 w918 w989 w1017]
      tunnel: w16 -> [w66 w92 w118 w144 w170 w196 w222 w256 w282 w308 w333 w357 w383 w409 w456 w482 w513 w554 w594 w662 _ _ w820 w848 w883 w917 w988 w1016]
      tunnel: w15 -> [w65 w91 w117 w143 w169 w195 w221 w255 w281 w307 w332 w356 w382 w408 w455 w483 w512 w553 w593 w661 w709 w768 w819 w847 w882 w916 w987 w1015]
      tunnel: [w65 w91 w117 w143 w169 w195 w221 w255 w281 w307 w332 w356 w382 w408 w455 _ w512 w553 w593 w661 w709 w769 w819 w847 w882 w916 w987 w1015] -> w14
      tunnel: [w66 w92 w118 w144 w170 w196 w222 w256 w282 w308 w333 w357 w383 w409 w456 w482 w513 w554 w594 w662 w710 _ w820 w848 w883 w917 w988 w1016] -> w13
      tunnel: [_ _ _ _ _ _ _ _ _ _ _ _ _ _ _ w483 _ _ _ _ _ _ _ _ _ _ _ _] -> _
      frame "Initialize" {
        w70 = FALSE ("P1")
        # "Get Device Handle !"
        # "Switch Initialize ....."
        n10 = local write "Export"(w70) -> ()
        n11 = local write "P4"(w70) -> ()
        n12 = local write "P1"(w70) -> ()
        n13 = local write "Start"(w70) -> ()
        n14 = local write "EXIT"(w70) -> ()
        n15 = call "Open.vi"() -> ("Handle Number"=w78:i32)  [unwired: 10 in, 1 out]
        "Handle Number" <- w78
        n16 = local write "P2"(w70) -> ()
        n17 = local write "P5"(w70) -> ()
        n18 = local write "Correction"(w70) -> ()
        n19 = local write "Stop"(w70) -> ()
        n20 = local write "P3"(w70) -> ()
        n21 = local write "P6"(w70) -> ()
        n22 = local write "Auto-Sweep"(w70) -> ()
        n23 = local write "P7"(w70) -> ()
        n24 = Build Array (concatenate)(w76, "ActiveSwitch") -> (w75:string[])
        n25 = local write "P8"(w70) -> ()
      }
      frame "ActiveSwitch" {
        w96 = T2."Enabled" ("無効")
        # "Set Active Mode to the Switch"
        n26 = property on="P1" class="Bool (strict)"("DisabledEnum"=w96) -> ()  [unwired: 2 in, 2 out]
        n27 = property on="P5" class="Bool (strict)"("DisabledEnum"=w96) -> ()  [unwired: 2 in, 2 out]
        n28 = property on="P7" class="Bool (strict)"("DisabledEnum"=w96) -> ()  [unwired: 2 in, 2 out]
        n29 = property on="P2" class="Bool (strict)"("DisabledEnum"=w96) -> ()  [unwired: 2 in, 2 out]
        n30 = property on="P6" class="Bool (strict)"("DisabledEnum"=w96) -> ()  [unwired: 2 in, 2 out]
        n31 = property on="P8" class="Bool (strict)"("DisabledEnum"=w96) -> ()  [unwired: 2 in, 2 out]
        n32 = property on="P3" class="Bool (strict)"("DisabledEnum"=w96) -> ()  [unwired: 2 in, 2 out]
        n33 = property on="EXIT" class="Bool (strict)"("DisabledEnum"=w96) -> ()  [unwired: 2 in, 2 out]
        n34 = property on="Export" class="Bool (strict)"("DisabledEnum"=w96) -> ()  [unwired: 2 in, 2 out]
        n35 = property on="P4" class="Bool (strict)"("DisabledEnum"=w96) -> ()  [unwired: 2 in, 2 out]
        n36 = case shown="True" w98 {
          tunnel: w96 -> [_ w116]
          frame False {
          }
          frame True {
            n37 = property on="Start" class="Bool (strict)"("DisabledEnum"=w116) -> ()  [unwired: 2 in, 2 out]
          }
        }
      }
      frame "LockSwitch" {
        w122 = T2."Disabled and Grayed Out" ("無効")
        # "Set Lock Mode to the Switch"
        n38 = property on="P1" class="Bool (strict)"("DisabledEnum"=w122) -> ()  [unwired: 2 in, 2 out]
        n39 = property on="P5" class="Bool (strict)"("DisabledEnum"=w122) -> ()  [unwired: 2 in, 2 out]
        n40 = property on="P7" class="Bool (strict)"("DisabledEnum"=w122) -> ()  [unwired: 2 in, 2 out]
        n41 = property on="P2" class="Bool (strict)"("DisabledEnum"=w122) -> ()  [unwired: 2 in, 2 out]
        n42 = property on="P6" class="Bool (strict)"("DisabledEnum"=w122) -> ()  [unwired: 2 in, 2 out]
        n43 = property on="P8" class="Bool (strict)"("DisabledEnum"=w122) -> ()  [unwired: 2 in, 2 out]
        n44 = property on="P3" class="Bool (strict)"("DisabledEnum"=w122) -> ()  [unwired: 2 in, 2 out]
        n45 = property on="EXIT" class="Bool (strict)"("DisabledEnum"=w122) -> ()  [unwired: 2 in, 2 out]
        n46 = property on="Export" class="Bool (strict)"("DisabledEnum"=w122) -> ()  [unwired: 2 in, 2 out]
        n47 = property on="P4" class="Bool (strict)"("DisabledEnum"=w122) -> ()  [unwired: 2 in, 2 out]
        n48 = case shown="True" w124 {
          tunnel: w122 -> [_ w142]
          frame False {
          }
          frame True {
            n49 = property on="Start" class="Bool (strict)"("DisabledEnum"=w142) -> ()  [unwired: 2 in, 2 out]
          }
        }
      }
      frame "SetPower" {
        # "Set power of the PMT-Module"
        n50 = local read "P1"() -> (w154:bool)
        n51 = Boolean To (0,1)(Boolean=w154) -> (0, 1=w153:i16)
        n52 = To Long Integer(number=w153) -> (32bit integer=w152:i32)
        n53 = call "Set HV.vi"("HV"=w152, "handle"=w155) -> ()  [unwired: 8 in, 2 out]
      }
      frame "SetIT" {
        # "Set internal time ....."
        n54 = local read "IT"() -> (w179:i32)
        n55 = To Long Integer(number=w179) -> (32bit integer=w180:i32)
        n56 = call "Set IT.vi"("IT"=w180, "handle"=w181) -> ()  [unwired: 8 in, 2 out]
        n57 = local write "P3"(FALSE ("P3")) -> ()
      }
      frame "SetRN" {
        # "Set read number ....."
        n58 = local read "RN"() -> (w205:i32)
        n59 = To Long Integer(number=w205) -> (32bit integer=w206:i32)
        n60 = call "Set RN.vi"("RN"=w206, "handle"=w207) -> ()  [unwired: 8 in, 2 out]
        n61 = local write "P5"(FALSE ("P3")) -> ()
      }
      frame "SetStepProp" {
        # "Set Step SIze properties....."
        n62 = stacked-sequence {
          frame #0 {
            n63 = local read "WT"() -> (w246:i32)
            n64 = local read "ES"() -> (w245:i32)
            n65 = local read "SS"() -> (w247:i32)
            n66 = local read "EP"() -> (w248:i32)
            n67 = local read "SP"() -> (w249:i32)
            n68 = local write "SSD"(w247) -> ()
            n69 = local write "WTD"(w246) -> ()
            n70 = local write "ESD"(w245) -> ()
            n71 = local write "SPD"(w249) -> ()
            n72 = local write "EPD"(w248) -> ()
          }
          frame #1 {
            n73 = local read "EP"() -> (w254:i32)
            n74 = local read "SS"() -> (w253:i32)
            n75 = local read "ES"() -> (w251:i32)
            n76 = Divide(x=w254, y=w253) -> (x/y=w252:dbl)
            n77 = Add(x=w252, y=w251) -> (x+y=w250:dbl)
            n78 = local write "SND"(w250) -> ()
          }
        }
        n79 = local write "P7"(FALSE) -> ()
      }
      frame "ReadPower" {
        # "Read power flag of the PMT-Module"
        n80 = local read "PowerD"() -> (w267:i32)
        n81 = call "Read HV.vi"("HV"=w267, "handle"=w266) -> ("HV out"=w265:i32)  [unwired: 7 in, 2 out]
        n82 = local write "PowerD"(w265) -> ()
        n83 = local write "P2"(FALSE ("P2")) -> ()
      }
      frame "ReadIT" {
        # "Read internal time of the PMT-Module"
        n84 = local read "ITD"() -> (w293:i32)
        n85 = call "Read IT.vi"("IT"=w293, "handle"=w292) -> ("IT out"=w291:i32)  [unwired: 7 in, 2 out]
        n86 = local write "ITD"(w291) -> ()
        n87 = local write "P4"(FALSE ("P4")) -> ()
      }
      frame "ReadRN" {
        # "Read data read number of the PMT-Module"
        n88 = local read "RND"() -> (w319:i32)
        n89 = call "Read RN.vi"("RN"=w319, "handle"=w318) -> ("RN out"=w316:i32)  [unwired: 7 in, 2 out]
        n90 = local write "RND"(w316) -> ()
        n91 = local write "P6"(FALSE ("P4")) -> ()
      }
      frame "ReadSN" {
        # "Read data sweep number of the Motorized stage"
        n92 = Increment(x=w334) -> (x+1=w335:i32)
        n93 = local write "SN"(w335) -> ()
      }
      frame "CountStart" {
        # "Conter Start!"
        n94 = local read "Correction"() -> (w365:bool)
        n95 = Boolean To (0,1)(Boolean=w365) -> (0, 1=w367:i16)
        n96 = To Long Integer(number=w367) -> (32bit integer=w366:i32)
        n97 = call "Count Start.vi"("Correction"=w366, "handle"=w368) -> ()  [unwired: 8 in, 2 out]
      }
      frame "CountStop" {
        w384 = FALSE ("Start")
        # "Add Auto Sweep button local variable here"
        # "Conter Stop!"
        n98 = local write "Auto-Sweep"(w384) -> ()
        n99 = local write "Stop"(w384) -> ()
        n100 = local write "Start"(w384) -> ()
        n101 = call "Count Stop.vi"("handle"=w395) -> ()  [unwired: 9 in, 2 out]
        n102 = Build Array (concatenate)(w393, "ActiveSwitch") -> (w392:string[])
      }
      frame "ReadData" {
        # "Read Data...."
        n103 = stacked-sequence {
          seq-local: [_ w441 _] -> [_ _ w451]
          seq-local: [_ w440 _] -> [_ _ w452]
          tunnel: w420 -> [_ w446 _]
          tunnel: w419 -> [_ _ w454]
          tunnel: [_ _ w453] -> w418
          tunnel: [_ w436 _] -> w417
          tunnel: w416 -> [_ w439 _]
          frame #0 {
            # "DB Clear!"
            n104 = Initialize Array(u32 0, 16 ("次元サイズ")) -> (w433:u32[])
            n105 = local write "DB"(w433) -> ()
          }
          frame #1 {
            n106 = local read "OLD"() -> (w443:i32)
            n107 = local read "GN"() -> (w445:i32)
            n108 = local read "DB"() -> (w444:u32[])
            n109 = call "Read Data.vi"("OLD"=w443, "DataBuf"=w444, "GateNum"=w445, "handle"=w446) -> ("OLD out"=w442:i32, "DataBuf out"=w440:u32[], "GateNum out"=w438:i32, "function return"=w441:u32)  [unwired: 3 in, 1 out]
            n110 = local write "OLD"(w442) -> ()
            n111 = local write "GN"(w438) -> ()
            n112 = local write "DB"(w440) -> ()
            n113 = Build Array(w438) -> (w437:i32[])
            n114 = Build Array (concatenate)(w439, w437) -> (w436:i32[])
          }
          frame #2 {
            # "Check Over Rang !"
            # "ADD Data DIM"
            # "Pickup Tans Data!"
            n115 = To Long Integer(number=w451) -> (32bit integer=w449:i32)
            n116 = local read "OLD"() -> (w448:i32)
            n117 = Array Subset(array=w452, length=w449) -> (w450:u32[])  [unwired: 1 in]
            n118 = Not Equal To 0?(x=w448) -> (x != 0?=w447:bool)
            n119 = local write "OVL"(w447) -> ()
            n120 = Build Array (concatenate)(w454, w450) -> (w453:u32[])
            n121 = local write "Graph"(w453) -> ()
          }
        }
      }
      frame "AutoReadData" {
        # "Read Data...."
        n122 = stacked-sequence {
          tunnel: w459 -> [w481]
          tunnel: [w480] -> w458
          tunnel: w457 -> [w479]
          frame #0 {
            n123 = Build Array (concatenate)(w479, w481) -> (w480:dbl[])
            n124 = local write "Sweep Graph"(w480) -> ()
          }
        }
      }
      frame "CountInit" {
        w492 = 0
        # "Auto"
        # "Clear Data DIM !"
        n125 = Initialize Array(w492, w492) -> (w490:i32[])
        n126 = Build Array("LockSwitch", "ReadRN", "CountStart", "ReadData", "CheckNumber") -> (w493:string[])
        n127 = Build Array (concatenate)(w499, w493) -> (w498:string[])
      }
      frame "AutoCount|nit!" {
        w527 = 0
        # "Clear Data DIM !"
        n128 = local read "SND"() -> (w514:i32)
        n129 = local read "SN"() -> (w519:i32)
        n130 = Increment(x=w514) -> (x+1=w515:i32)
        n131 = Initialize Array(w527, w527) -> (w526:i32[])
        n132 = Less?(x=w519, y=w515) -> (x < y?=w518:bool)
        n133 = case shown="True" w518 {
          tunnel: w517 -> [w543 w546]
          tunnel: [w541 w545] -> w516
          frame False {
            n134 = Build Array("AutoReadData", "AutoCheckNumber") -> (w542:string[])
            n135 = Build Array (concatenate)(w543, w542) -> (w541:string[])
          }
          frame True {
            n136 = Build Array("LockSwitch", "ReadRN", "CountStart", "ReadData", "AutoCheckNumber") -> (w552:string[])
            n137 = Build Array (concatenate)(w546, w552) -> (w545:string[])
          }
        }
      }
      frame "CheckNumber" {
        # "Add append"
        # "Add Case Strucutre outside\nsimilar to GN,"
        # "Check RN and Data lenbgth,Stop Switch ......"
        n138 = local read "Stop"() -> (w563:bool)
        n139 = local read "GN"() -> (w564:i32)
        n140 = Decrement(x=w566) -> (x-1=w565:i32)
        n141 = Less?(x=w564, y=w565) -> (x < y?=w570:bool)
        n142 = case shown="False" w570 {
          tunnel: [w585 w587] -> w567
          tunnel: w563 -> [_ w586]
          frame False {
            # "\"MotorJog\"; here"
            # "Move \"Active Swith\" to False Condition of Position Number"
            # "Add \"AutoExport Run\" here"
            n143 = local write "Start"(FALSE ("Start")) -> ()
            n144 = Build Array("CountStop", "ActiveSwitch") -> (w585:string[])
          }
          frame True {
            n145 = case shown="False" w586 {
              tunnel: [w589 w591] -> w587
              frame False {
                n146 = Build Array("ReadData", "CheckNumber") -> (w589:string[])
              }
              frame True {
                n147 = Build Array("CountStop") -> (w591:string[])
              }
            }
          }
        }
        n148 = Build Array (concatenate)(w568, w567) -> (w569:string[])
      }
      frame "AutoCheckNumber" {
        # "Add append"
        # "Add Case Strucutre outside\nsimilar to GN,"
        # "Check RN and Data lenbgth,Stop Switch ......"
        n149 = local read "Stop"() -> (w606:bool)
        n150 = local read "SND"() -> (w595:i32)
        n151 = local read "SN"() -> (w599:i32)
        n152 = Less?(x=w599, y=w595) -> (x < y?=w598:bool)
        n153 = case shown="False" w598 {
          tunnel: [w623 w633] -> w608
          tunnel: w607 -> [_ w632]
          tunnel: w606 -> [_ w629]
          tunnel: [TRUE w628] -> w601
          frame False {
            w627 = FALSE ("Start")
            n154 = local write "Auto-Sweep"(w627) -> ()
            n155 = local write "Start"(w627) -> ()
            n156 = Build Array("CountStop", "AutoExportSweep", "ActiveSwitch") -> (w623:string[])
          }
          frame True {
            n157 = local read "GN"() -> (w630:i32)
            n158 = Decrement(x=w632) -> (x-1=w631:i32)
            n159 = Less?(x=w630, y=w631) -> (x < y?=w634:bool)
            n160 = case shown="False" w634 {
              tunnel: [w636 w652] -> w633
              tunnel: w629 -> [w637 w651]
              tunnel: [w635 w650] -> w628
              frame False {
                # "\"MotorJog\"; here"
                # "Move \"Active Swith\" to False Condition of Position Number"
                # "Add \"AutoExport Run\" here"
                n161 = case shown="False" w637 {
                  tunnel: [w643 w648] -> w636
                  tunnel: [FALSE TRUE] -> w635
                  frame False {
                    n162 = Build Array("CountStop", "AutoExportRun", "AutoReadData", "ReadSN", "MotorJog", "AutoCount|nit!") -> (w643:string[])
                  }
                  frame True {
                    n163 = local write "Auto-Sweep"(TRUE) -> ()
                    n164 = Build Array("CountStop") -> (w648:string[])
                  }
                }
              }
              frame True {
                n165 = case shown="False" w651 {
                  tunnel: [w655 w659] -> w652
                  tunnel: [FALSE TRUE] -> w650
                  frame False {
                    n166 = Build Array("ReadData", "AutoCheckNumber") -> (w655:string[])
                  }
                  frame True {
                    n167 = Build Array("CountStop") -> (w659:string[])
                    n168 = local write "Auto-Sweep"(TRUE) -> ()
                  }
                }
              }
            }
          }
        }
        n169 = Build Array (concatenate)(w609, w608) -> (w610:string[])
      }
      frame "Export" {
        # "For Auto Export also add mean waveform"
        # "Get mean Data into 1D array Shift register for waveform"
        # "Gate Number is just number of count measurements"
        # "time...using array size"
        # "time...using array size"
        n170 = Array Size(array=w677) -> (size(s)=w689:i32)
        n171 = for {
          N: w689 -> [_]
          tunnel: [w704] -> w676 mode=indexing
          i -> [w706]
          n172 = local read "ITD"() -> (w708:i32)
          n173 = Add(x=1, y=w706) -> (x+y=w707:i32)
          n174 = Multiply(x=w708, y=w707) -> (x*y=w704:i32)
        }
        n175 = call <vilib>:"Std Deviation and Variance.vi"("X"=w677) -> ("mean"=w670:dbl, "standard deviation"=w669:dbl)  [unwired: 1 in, 1 out]
        n176 = Build Array(w670, w669) -> (w668:dbl[])
        n177 = Build Array(w672, w676, w677) -> (w687:u32[][])
        n178 = call-poly <vilib>:"Write Delimited Spreadsheet.vi"("1D data"=string[] ["Gate  No.", "Time [ms]", "Counts"], "append to file? (new file:F)"=FALSE, "transpose? (no:F)"=FALSE) -> ("new file path (Not A Path if cancelled)"=w686:path)  [unwired: 11 in, 1 out]
        n179 = call-poly <vilib>:"Write Delimited Spreadsheet.vi"("file path (dialog if empty)"=w686, "2D data"=w687, "append to file? (new file:F)"=TRUE, "transpose? (no:F)"=TRUE) -> ("new file path (Not A Path if cancelled)"=w682:path)  [unwired: 10 in, 1 out]
        n180 = call-poly <vilib>:"Write Delimited Spreadsheet.vi"("file path (dialog if empty)"=w682, "1D data"=string[] ["Mean", "Std. Dev."], "append to file? (new file:F)"=TRUE, "transpose? (no:F)"=FALSE) -> ("new file path (Not A Path if cancelled)"=w678:path)  [unwired: 10 in, 1 out]
        n181 = call-poly <vilib>:"Write Delimited Spreadsheet.vi"("file path (dialog if empty)"=w678, "1D data"=w668, "append to file? (new file:F)"=TRUE, "transpose? (no:F)"=FALSE) -> ()  [unwired: 10 in, 2 out]
        n182 = local write "Export"(FALSE) -> ()
      }
      frame "AutoExportRun" {
        # "For Auto Export also add mean waveform"
        # "Get mean Data into 1D array Shift register for waveform"
        # "Gate Number is just number of count measurements"
        # "time...using array size"
        # "time...using array size"
        n183 = Array Size(array=w731) -> (size(s)=w743:i32)
        n184 = for {
          N: w743 -> [_]
          tunnel: [w763] -> w730 mode=indexing
          i -> [w765]
          n185 = local read "ITD"() -> (w767:i32)
          n186 = Add(x=1, y=w765) -> (x+y=w766:i32)
          n187 = Multiply(x=w767, y=w766) -> (x*y=w763:i32)
        }
        n188 = flat-sequence {
          tunnel: w715 -> [w762]
          tunnel: [w758] -> w714
          frame #0 {
            n189 = local read "SS"() -> (w761:i32)
            n190 = Multiply(x=w762, y=w761) -> (x*y=w759:i32)
            n191 = local read "SP"() -> (w760:i32)
            n192 = Add(x=w760, y=w759) -> (x+y=w758:i32)
          }
        }
        n193 = call <vilib>:"Std Deviation and Variance.vi"("X"=w731) -> ("mean"=w721:dbl, "standard deviation"=w710:dbl)  [unwired: 1 in, 1 out]
        n194 = Build Array(w721, w710) -> (w724:dbl[])
        n195 = Number To Decimal String(number=w714) -> (decimal integer string=w713:string)  [unwired: 1 in]
        n196 = Build Array(w726, w730, w731) -> (w741:u32[][])
        n197 = Build Array (concatenate)(string[] ["Angle (deg)"], w713) -> (w711:string[])
        n198 = call-poly <vilib>:"Write Delimited Spreadsheet.vi"("file path (dialog if empty)"=w719, "1D data"=w711, "append to file? (new file:F)"=TRUE, "transpose? (no:F)"=FALSE) -> ("new file path (Not A Path if cancelled)"=w718:path)  [unwired: 10 in, 1 out]
        n199 = call-poly <vilib>:"Write Delimited Spreadsheet.vi"("file path (dialog if empty)"=w718, "1D data"=string[] ["Gate  No.", "Time [ms]", "Counts"], "append to file? (new file:F)"=TRUE, "transpose? (no:F)"=FALSE) -> ("new file path (Not A Path if cancelled)"=w740:path)  [unwired: 10 in, 1 out]
        n200 = call-poly <vilib>:"Write Delimited Spreadsheet.vi"("file path (dialog if empty)"=w740, "2D data"=w741, "append to file? (new file:F)"=TRUE, "transpose? (no:F)"=TRUE) -> ("new file path (Not A Path if cancelled)"=w736:path)  [unwired: 10 in, 1 out]
        n201 = call-poly <vilib>:"Write Delimited Spreadsheet.vi"("file path (dialog if empty)"=w736, "1D data"=string[] ["Mean", "Std. Dev."], "append to file? (new file:F)"=TRUE, "transpose? (no:F)"=FALSE) -> ("new file path (Not A Path if cancelled)"=w732:path)  [unwired: 10 in, 1 out]
        n202 = call-poly <vilib>:"Write Delimited Spreadsheet.vi"("file path (dialog if empty)"=w732, "1D data"=w724, "append to file? (new file:F)"=TRUE, "transpose? (no:F)"=FALSE) -> ("new file path (Not A Path if cancelled)"=w723:path)  [unwired: 10 in, 1 out]
        n203 = local write "Export"(FALSE) -> ()
      }
      frame "AutoExportSweep" {
        w771 = 0
        w770 = 0.0
        # "For Auto Export also add mean waveform"
        # "Get mean Data into 1D array Shift register for waveform"
        # "Gate Number is just number of count measurements"
        # "time...using array size"
        # "time...using array size"
        n204 = Array Size(array=w774) -> (size(s)=w799:i32)
        n205 = for {
          N: w799 -> [_]
          tunnel: [w817] -> w786 mode=indexing
          i -> [w814]
          n206 = local read "SS"() -> (w818:i32)
          n207 = Multiply(x=w818, y=w814) -> (x*y=w815:i32)
          n208 = local read "SP"() -> (w816:i32)
          n209 = Add(x=w816, y=w815) -> (x+y=w817:i32)
        }
        n210 = Initialize Array(w770, w771) -> (w772:dbl[])
        n211 = Initialize Array(w770, w771) -> (w769:dbl[])
        n212 = call <vilib>:"Std Deviation and Variance.vi"("X"=w774) -> ("mean"=w775:dbl, "standard deviation"=w780:dbl)  [unwired: 1 in, 1 out]
        n213 = Build Array(w775, w780) -> (w779:dbl[])
        n214 = Build Array(w786, w774, w768) -> (w797:dbl[][])
        n215 = call-poly <vilib>:"Write Delimited Spreadsheet.vi"("file path (dialog if empty)"=w776, "1D data"=string[] ["Angle Itr.", "Counts Mean", ""], "append to file? (new file:F)"=TRUE, "transpose? (no:F)"=FALSE) -> ("new file path (Not A Path if cancelled)"=w796:path)  [unwired: 10 in, 1 out]
        n216 = call-poly <vilib>:"Write Delimited Spreadsheet.vi"("file path (dialog if empty)"=w796, "2D data"=w797, "append to file? (new file:F)"=TRUE, "transpose? (no:F)"=TRUE) -> ("new file path (Not A Path if cancelled)"=w792:path)  [unwired: 10 in, 1 out]
        n217 = call-poly <vilib>:"Write Delimited Spreadsheet.vi"("file path (dialog if empty)"=w792, "1D data"=string[] ["Mean", "Std. Dev."], "append to file? (new file:F)"=TRUE, "transpose? (no:F)"=FALSE) -> ("new file path (Not A Path if cancelled)"=w788:path)  [unwired: 10 in, 1 out]
        n218 = call-poly <vilib>:"Write Delimited Spreadsheet.vi"("file path (dialog if empty)"=w788, "1D data"=w779, "append to file? (new file:F)"=TRUE, "transpose? (no:F)"=FALSE) -> ("new file path (Not A Path if cancelled)"=w778:path)  [unwired: 10 in, 1 out]
        n219 = local write "Export"(FALSE) -> ()
      }
      frame "AutoSweep" {
        w823 = 0
        # "1. Create a file path (Send two strings, \"SetPosition\" and \"AutoCount|nit!\")\n2. Send to \"SetPosition\"\n2.1. Will create a Position Number Shift register\n2.2. Move stage to initial position, allow time to complete movement or add delay\n3. Send to \"AutoCount|nit!\"\n3.1. \"AutoCount|nit!\" is clone of \"Count|nit!\" but sends to \"AutoCheckNumber\", not \"CheckNumber\n3.1.1. \"AutoCheckNumber\" will check if end position, or run condition is met then send \"CountStop\" and \"ActiveSwitch\"\n3.1.2. \"AutoCheck Number\" will allow \"CountStop\" to be sent via Stop Boolean\n3.1.3. \"AutoCheckNumber\" will upon END of one run will run \"AutoExportRun\" to set file path\n3.1.3.1. \"AutoExportRun\" will add a data point to Mean Waveform after Count Stop\n3.1.4. \"AutoCheckNumber\" will upon END of sweep will run \"AutoExportSweep\" then issue \"ActiveSwitch\"\n3.1.4.1. \"AutoExportSweep\" will append final Mean Sweep waveform to file path before \"CountStop\";\"ActiveSwitch\"\n4. If End condition not met; \"MotorJog\"; \"AutoCount|nit!\"....repeats\n4.1. Will move to next position by set increment, with .net code, add delay to allow it to arrive at position"
        # "Create a File path here\nSend switch case string \"SetPosition\", which has a position number switch register"
        # "1.Position Set, create a file path\n2. Count|nit!---duplicate and create auto counter, add read sweep data for auto read\n2.0.1Checknumber end, change active switch to Auto export\n3. Auto Export ... need to make \n3.0.2Auto Export end, send to read sweep data (mean, stdev for per sweep)\n3.Export\n4.check end position, check end condition met\n5.met>end;not end >continue\n6. Jog motor\n7.repeat from 2."
        # "Create Motor Controls for setting Homing, Step size for angle, idle time(if required),"
        n220 = local write "SN"(w823) -> ()
        n221 = call-poly <vilib>:"Write Delimited Spreadsheet.vi"("append to file? (new file:F)"=FALSE) -> ("new file path (Not A Path if cancelled)"=w822:path)  [unwired: 13 in, 1 out]
        n222 = Build Array("SetPosition", "AutoCount|nit!") -> (w828:string[])
        n223 = Build Array (concatenate)(w826, w828) -> (w825:string[])
      }
      frame "MotorJog" {
        # "Move position by set increment"
        # "Add a test Jog?"
        # "Put thor labs net code here"
        n224 = stacked-sequence {
          tunnel: w854 -> [w876 w881]
          frame #0 {
            n225 = local read "SSD"() -> (w875:i32)
            n226 = invoke class="KCubeDCServo" method="MoveRelative"(reference=w876, "direction"=1, "stepSize"=w875, "waitTimeout"=0) -> ()  [unwired: 2 in, 6 out]
            n227 = local read "WT"() -> (w873:i32)
            n228 = Wait (ms)(milliseconds to wait=w873) -> ()  [unwired: 1 out]
          }
          frame #1 {
            n229 = invoke class="KCubeDCServo" method="GetPositionCounter"(reference=w881) -> ("GetPositionCounter"=w879:i32)  [unwired: 2 in, 2 out]
            n230 = Divide(x=w879, y=1919.6418578623338) -> (x/y=w877:dbl)
            n231 = Wait (ms)(milliseconds to wait=50) -> ()  [unwired: 1 out]
            n232 = local write "PC"(w877) -> ()
          }
        }
        n233 = local write "P8"(FALSE) -> ()
      }
      frame "SetPosition" {
        n234 = stacked-sequence {
          tunnel: w888 -> [w907 w910 w915]
          frame #0 {
            n235 = local read "SPD"() -> (w906:i32)
            n236 = invoke class="KCubeDCServo" method="SetMoveAbsolutePosition"(reference=w907, "position"=w906) -> ()  [unwired: 2 in, 4 out]
          }
          frame #1 {
            n237 = invoke class="KCubeDCServo" method="MoveAbsolute"(reference=w910, "waitTimeout"=0) -> ()  [unwired: 2 in, 4 out]
            n238 = local read "WT"() -> (w909:i32)
            n239 = Wait (ms)(milliseconds to wait=w909) -> ()  [unwired: 1 out]
          }
          frame #2 {
            n240 = invoke class="KCubeDCServo" method="GetPositionCounter"(reference=w915) -> ("GetPositionCounter"=w912:i32)  [unwired: 2 in, 2 out]
            n241 = Divide(x=w912, y=1919.6418578623338) -> (x/y=w911:dbl)
            n242 = local write "PC"(w911) -> ()
            n243 = Wait (ms)(milliseconds to wait=50) -> ()  [unwired: 1 out]
          }
        }
      }
      frame "", "Idle" {
        n244 = event shown="[12] \"Auto-Sweep\": Value Change" {
          selector: _ -> [_ _ _ _ _ _ _ _ _ _ _ _ _]
          dyn-events: _ -> [_ _ _ _ _ _ _ _ _ _ _ _ _]
          timeout: _ -> [_ _ _ _ _ _ _ _ _ _ _ _ _]
          tunnel: w929 -> [w944 w947 w950 w954 w958 w962 w966 w970 w973 w975 w978 w981 w984]
          tunnel: [w942 w946 w949 w953 w957 w961 w965 w969 w972 w974 w977 w980 w985] -> w927
          event Menu Selection (User) {
            n245 = event-data() -> ("ItemTag"=w943:string)  [unwired: 1 out]
            n246 = Build Array (concatenate)(w944, w943) -> (w942:string[])
          }
          event "EXIT": Value Change {
            n247 = event-data() -> ()  [unwired: 7 out]
            n248 = Build Array (concatenate)(w947, "Exit") -> (w946:string[])
          }
          event "P1": Value Change {
            n249 = event-data() -> ()  [unwired: 7 out]
            n250 = Build Array (concatenate)(w950, "SetPower") -> (w949:string[])
          }
          event "P2": Value Change {
            n251 = event-data() -> ()  [unwired: 7 out]
            n252 = Build Array (concatenate)(w954, "ReadPower") -> (w953:string[])
            n253 = Wait (ms)(milliseconds to wait=u32 200 ("ミリ秒待機時間")) -> ()  [unwired: 1 out]
          }
          event "P3": Value Change {
            n254 = event-data() -> ()  [unwired: 7 out]
            n255 = Build Array (concatenate)(w958, "SetIT") -> (w957:string[])
            n256 = Wait (ms)(milliseconds to wait=u32 200 ("ミリ秒待機時間")) -> ()  [unwired: 1 out]
          }
          event "P4": Value Change {
            n257 = event-data() -> ()  [unwired: 7 out]
            n258 = Build Array (concatenate)(w962, "ReadIT") -> (w961:string[])
            n259 = Wait (ms)(milliseconds to wait=u32 200 ("ミリ秒待機時間")) -> ()  [unwired: 1 out]
          }
          event "P5": Value Change {
            n260 = event-data() -> ()  [unwired: 7 out]
            n261 = Build Array (concatenate)(w966, "SetRN") -> (w965:string[])
            n262 = Wait (ms)(milliseconds to wait=u32 200 ("ミリ秒待機時間")) -> ()  [unwired: 1 out]
          }
          event "P6": Value Change {
            n263 = event-data() -> ()  [unwired: 7 out]
            n264 = Build Array (concatenate)(w970, "ReadRN") -> (w969:string[])
            n265 = Wait (ms)(milliseconds to wait=u32 200 ("ミリ秒待機時間")) -> ()  [unwired: 1 out]
          }
          event "Start": Value Change {
            n266 = event-data() -> ()  [unwired: 7 out]
            n267 = Build Array (concatenate)(w973, "CountInit") -> (w972:string[])
          }
          event "Export": Value Change {
            n268 = event-data() -> ()  [unwired: 7 out]
            n269 = Build Array (concatenate)(w975, "Export") -> (w974:string[])
          }
          event "P7": Value Change {
            n270 = event-data() -> ()  [unwired: 7 out]
            n271 = Build Array (concatenate)(w978, "SetStepProp") -> (w977:string[])
          }
          event "P8": Value Change {
            n272 = event-data() -> ()  [unwired: 7 out]
            n273 = Build Array (concatenate)(w981, "MotorJog") -> (w980:string[])
          }
          event "Auto-Sweep": Value Change {
            n274 = event-data() -> ()  [unwired: 7 out]
            n275 = Build Array (concatenate)(w984, "AutoSweep") -> (w985:string[])
            n276 = Wait (ms)(milliseconds to wait=200) -> ()  [unwired: 1 out]
          }
        }
        n277 = Build Array (concatenate)("", w927) -> (w926:string[])
      }
      frame "Error", Default {
        n278 = Concatenate Strings("Error  Case Name .....", "\r\n", w996) -> (w998:string)
        n279 = One Button Dialog(message=w998) -> (true=w997:bool)  [unwired: 1 out]
        n280 = stacked-sequence {
          tunnel: w997 -> [_]
          frame #0 {
            n281 = Stop() -> ()  [unwired: 1 out]
          }
        }
      }
      frame "Exit" {
        # "See you again ......"
        n282 = call "Close.vi"("Handle"=w1024) -> ()  [unwired: 9 in, 2 out]
      }
    }
    n283 = Divide(x=w18, y=1919.6418578623338) -> (x/y=w17:dbl)
    n284 = local write "PC"(w17) -> ()
    n285 = call "SM_CaseErase.vi"("Input"=w43) -> ("Output"=w42:string[])  [unwired: 10 out]
  }
  n286 = invoke class="KCubeDCServoControl" method="CloseDevice"(reference=w6) -> ()  [unwired: 2 in, 3 out]
